vi "4Pi Objective Lock.vi"(7 "Calling VI Ref":refnum<vi>) -> ()   [LabVIEW 2016]
uses:
  <vilib>/Utility/miscctls.llb/LVPointTypeDef.ctl
  4Pi Objective Lock Type Defs/4Pi Obj Lock - Notifier Type.ctl
  4Pi Objective Lock Type Defs/4Pi Obj Lock - Actions.ctl
  4Pi Objective Lock Type Defs/4Pi Obj Lock - Lock Settings.ctl
  Hardware Configuration/Hardware Configuration Controls/Device Type.ctl
  Hardware Configuration/Hardware Configuration Controls/Device Function.ctl
  4Pi Objective Lock Type Defs/4Pi Obj Lock - Camera Settings.ctl
  Device Library/Cameras/Camera Controls/Generic Camera ROI.ctl
  Device Library/Cameras/Camera Controls/Generic Camera Actions.ctl
  Device Library/Stages/Stages Controls/Stage Actions.ctl
  <vilib>/addons/control/pid/pid.llb/PID (DBL Array).vi
  <vilib>/addons/control/pid/NI_PID_pid.lvlib
panel:
  in  "Main Tab":T1(tab)
  out "Z Move":bool
  out "XY Move":bool
  out "Measured X Position (px)":dbl=1.0 format="%.3g"
  out "Measured Y Position (px)":dbl=1.0 format="%.3g"
  out "Measured sx/sy":dbl=1.0 format="%.3g"
  out "Target X Position (px)":dbl=1.0 format="%.3g"
  out "Target Y Position (px)":dbl=1.0 format="%.3g"
  out "Target sx/sy":dbl=1.0 format="%.3g"
  out "Z Axis Position (µm)":dbl=1.0 format="%.4g"
  out "Y Axis Position (µm)":dbl=1.0 format="%.2g"
  out "X Axis Position (µm)":dbl=1.0 format="%.2g"
  out "Z sx/sy Target and Fit Value":T2(graph)
  in  "Start Lock":bool
  out "Y Target and Fit Position (px)":T2(graph)
  out "X Target and Fit Position (px)":T2(graph)
  in  "Restart Lock":bool
  out "Fit Error":bool
  out "Move Limit Error":bool
  in  "Update Delay (ms)":i32=10
  in  "D (Derivative)":dbl
  in  "I (Integral)":dbl
  in  "P (Proportional)":dbl=2.0
  in  "Invert Z Axis":bool
  in  "XY Drift Threshold":dbl=0.05
  in  "Abort If Error":bool
  in  "Flip XY Axis":bool
  in  "Invert X Axis":bool
  in  "Invert Y Axis":bool
  in  "Z Stage Move Limit (µm)":dbl=5.0
  in  "Z Drift Threshold":dbl=0.05
  in  "XY Stage Move Limit (µm)":dbl=1.0
  in  "Frame Accumulations":u16=10
  in  "XY Correction Active":bool=TRUE
  in  "Z Correction Active":bool=TRUE
  in  "Set Camera ROI":bool
  in  "Save Lock Settings":bool
  in  "Quit":bool
  # "Z Drift Settings"
  # "Camera Setup"
  # "XY Drift Settings"
  # "PID Control Values"
  # "General Settings"
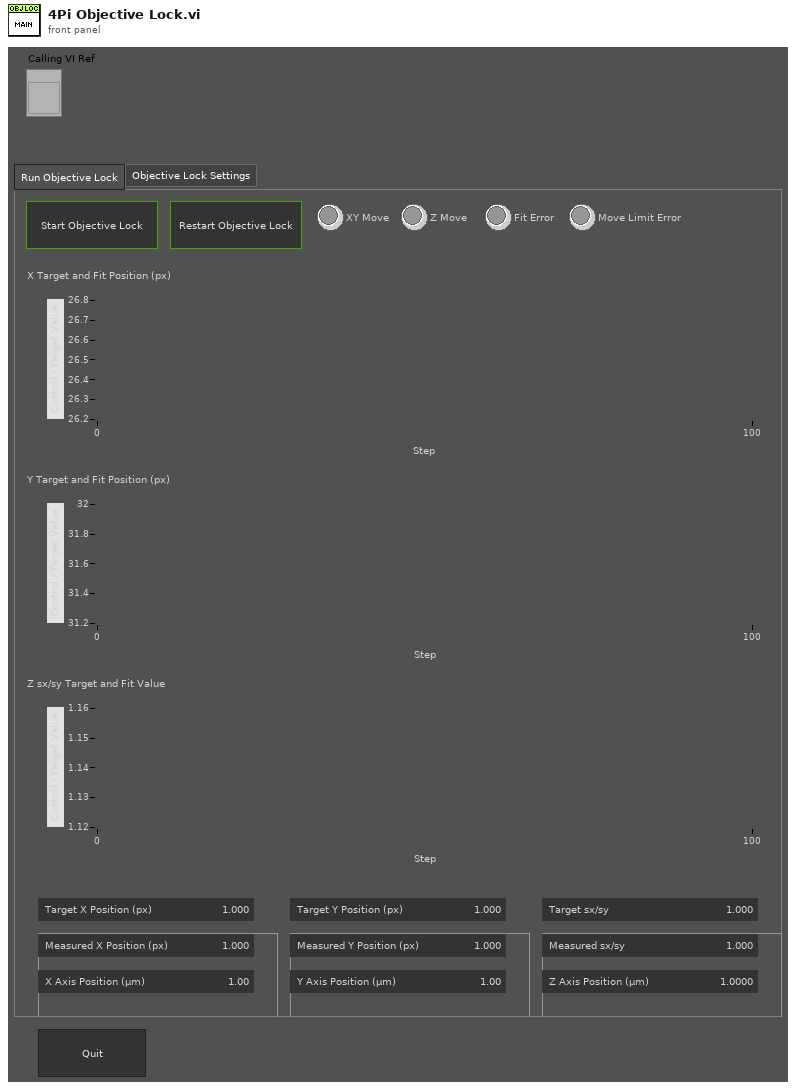
[diagram p1: front panel]
types:
  T1 = enum32{"Run Objective Lock", "Objective Lock Settings"}
  T2 = cluster{"Target 01":dbl, dbl, dbl, "Current 01":dbl}
  T3 = typedef "4Pi Obj Lock - Camera Settings.ctl" = cluster{"Exposure Time (s)":dbl, "H Offset":u16, "V Offset":u16, "H Width":u16, "V Width":u16}
  T4 = typedef "Device Function.ctl" = enum16{"Primary", "Secondary", "Overview", "Wide Field Drift Correction", "642 nm Excitation", "560 nm Excitation", "546 nm Excitation", "488 nm Excitation", "405 nm Excitation", "Objective Drift Correction", "4Pi Objective Lock", "Objective XY", "Objective Z", "Sample XY", "Sample Coarse Z", "Sample Z", "4Pi Lower", "4Pi Upper", "Adj Cavity", "Line Scanning", "Alert"}
  T5 = typedef "Device Type.ctl" = enum16{"AOTF", "Camera", "Deformable Mirror", "Laser", "Shutter", "Stage", "Waveform", "Email"}
  T6 = typedef "4Pi Obj Lock - Actions.ctl" = enum16{"Idle", "Start Lock", "Restart Lock", "Get Initial Position", "Get Current Position", "Check Drift", "Move XYZ", "Move XY", "Move Z", "Update Plots", "Delay", "Abort", "Exit Loop", "Quit"}
  T7 = typedef "4Pi Obj Lock - Lock Settings.ctl" = cluster{"Z Drift Threshold":dbl, "Z Stage Move Limit (µm)":dbl, "XY Drift Threshold":dbl, "XY Stage Move Limit (µm)":dbl, "Frame Accumulations":u16, "Abort If Error":bool, "Flip XY Axis":bool, "Invert X Axis":bool, "Invert Y Axis":bool, "Invert Z Axis":bool, "Z Correction Active":bool, "XY Correction Active":bool, "PID Values":dbl[], "Update Delay (ms)":i32}
  T8 = typedef "4Pi Obj Lock - Notifier Type.ctl" = cluster{"Actions":T6, "Z Drift Threshold":dbl, "Z Stage Move Limit (µm)":dbl, "XY Drift Threshold":dbl, "XY Stage Move Limit (µm)":dbl, "Frame Accumulations":u16, "Abort If Error":bool, "Z Correction Active":bool, "XY Correction Active":bool, "PID Values":dbl[], "Running?":bool, "Update Delay (ms)":i32}
  T9 = enum16{"Always On", "Always Off", "Off While Running"}
  T10 = typedef "LVPointTypeDef.ctl" = cluster{"Horizontal":i16, "Vertical":i16}
  T11 = typedef "Generic Camera Actions.ctl" = enum16{"Status", "Live Preview", "Capture", "Abort", "Set Exposure Time (s)", "Get Exposure Time (s)", "Record Settings", "Set ROI", "Get ROI", "Defect Correction On/Off", "Cooler On/Off", "Fan On/Off", "Quti"}
  T12 = typedef "Generic Camera ROI.ctl" = cluster{"H_Offset":u16, "V_Offset":u16, "H_Width":u16, "V_Width":u16}
  T13 = typedef "Stage Actions.ctl" = enum16{"Get Position", "MVR", "MOVE", "HALT", "ONTARGET", "ERROR", "REFERENCE", "INIT", "VELOCITY", "STATUS", "EXIT", "HOME", "ZEROPOS", "NANOPOS", "ANALOG", "QUIT"}
  T14 = enum32{"Invalid", "Standard", "Closed", "Hidden", "Minimized", "Maximized"}
  T15 = cluster{"Target 01":dbl, dbl, dbl, "Current 01":dbl}[]
  T16 = typedef "2D Gaussian - Best Fit Parameters.ctl" = cluster{"Amplitude":dbl, "X Position":dbl, "Y Position":dbl, "X Width":dbl, "Y Width":dbl, "Offset":dbl}
  T17 = cluster{"PID Values[0]":dbl, "PID Values[1]":dbl, "PID Values[2]":dbl}
  T18 = cluster{"PID Values[0]":dbl, "PID Values[1]":dbl, "PID Values[2]":dbl}[]
  T19 = typedef "LVRectTypeDef.ctl" = cluster{"Left":i16, "Top":i16, "Right":i16, "Bottom":i16}
  T20 = typedef "LVBoundsTypeDef.ctl" = cluster{"Width":u32, "Height":u32}
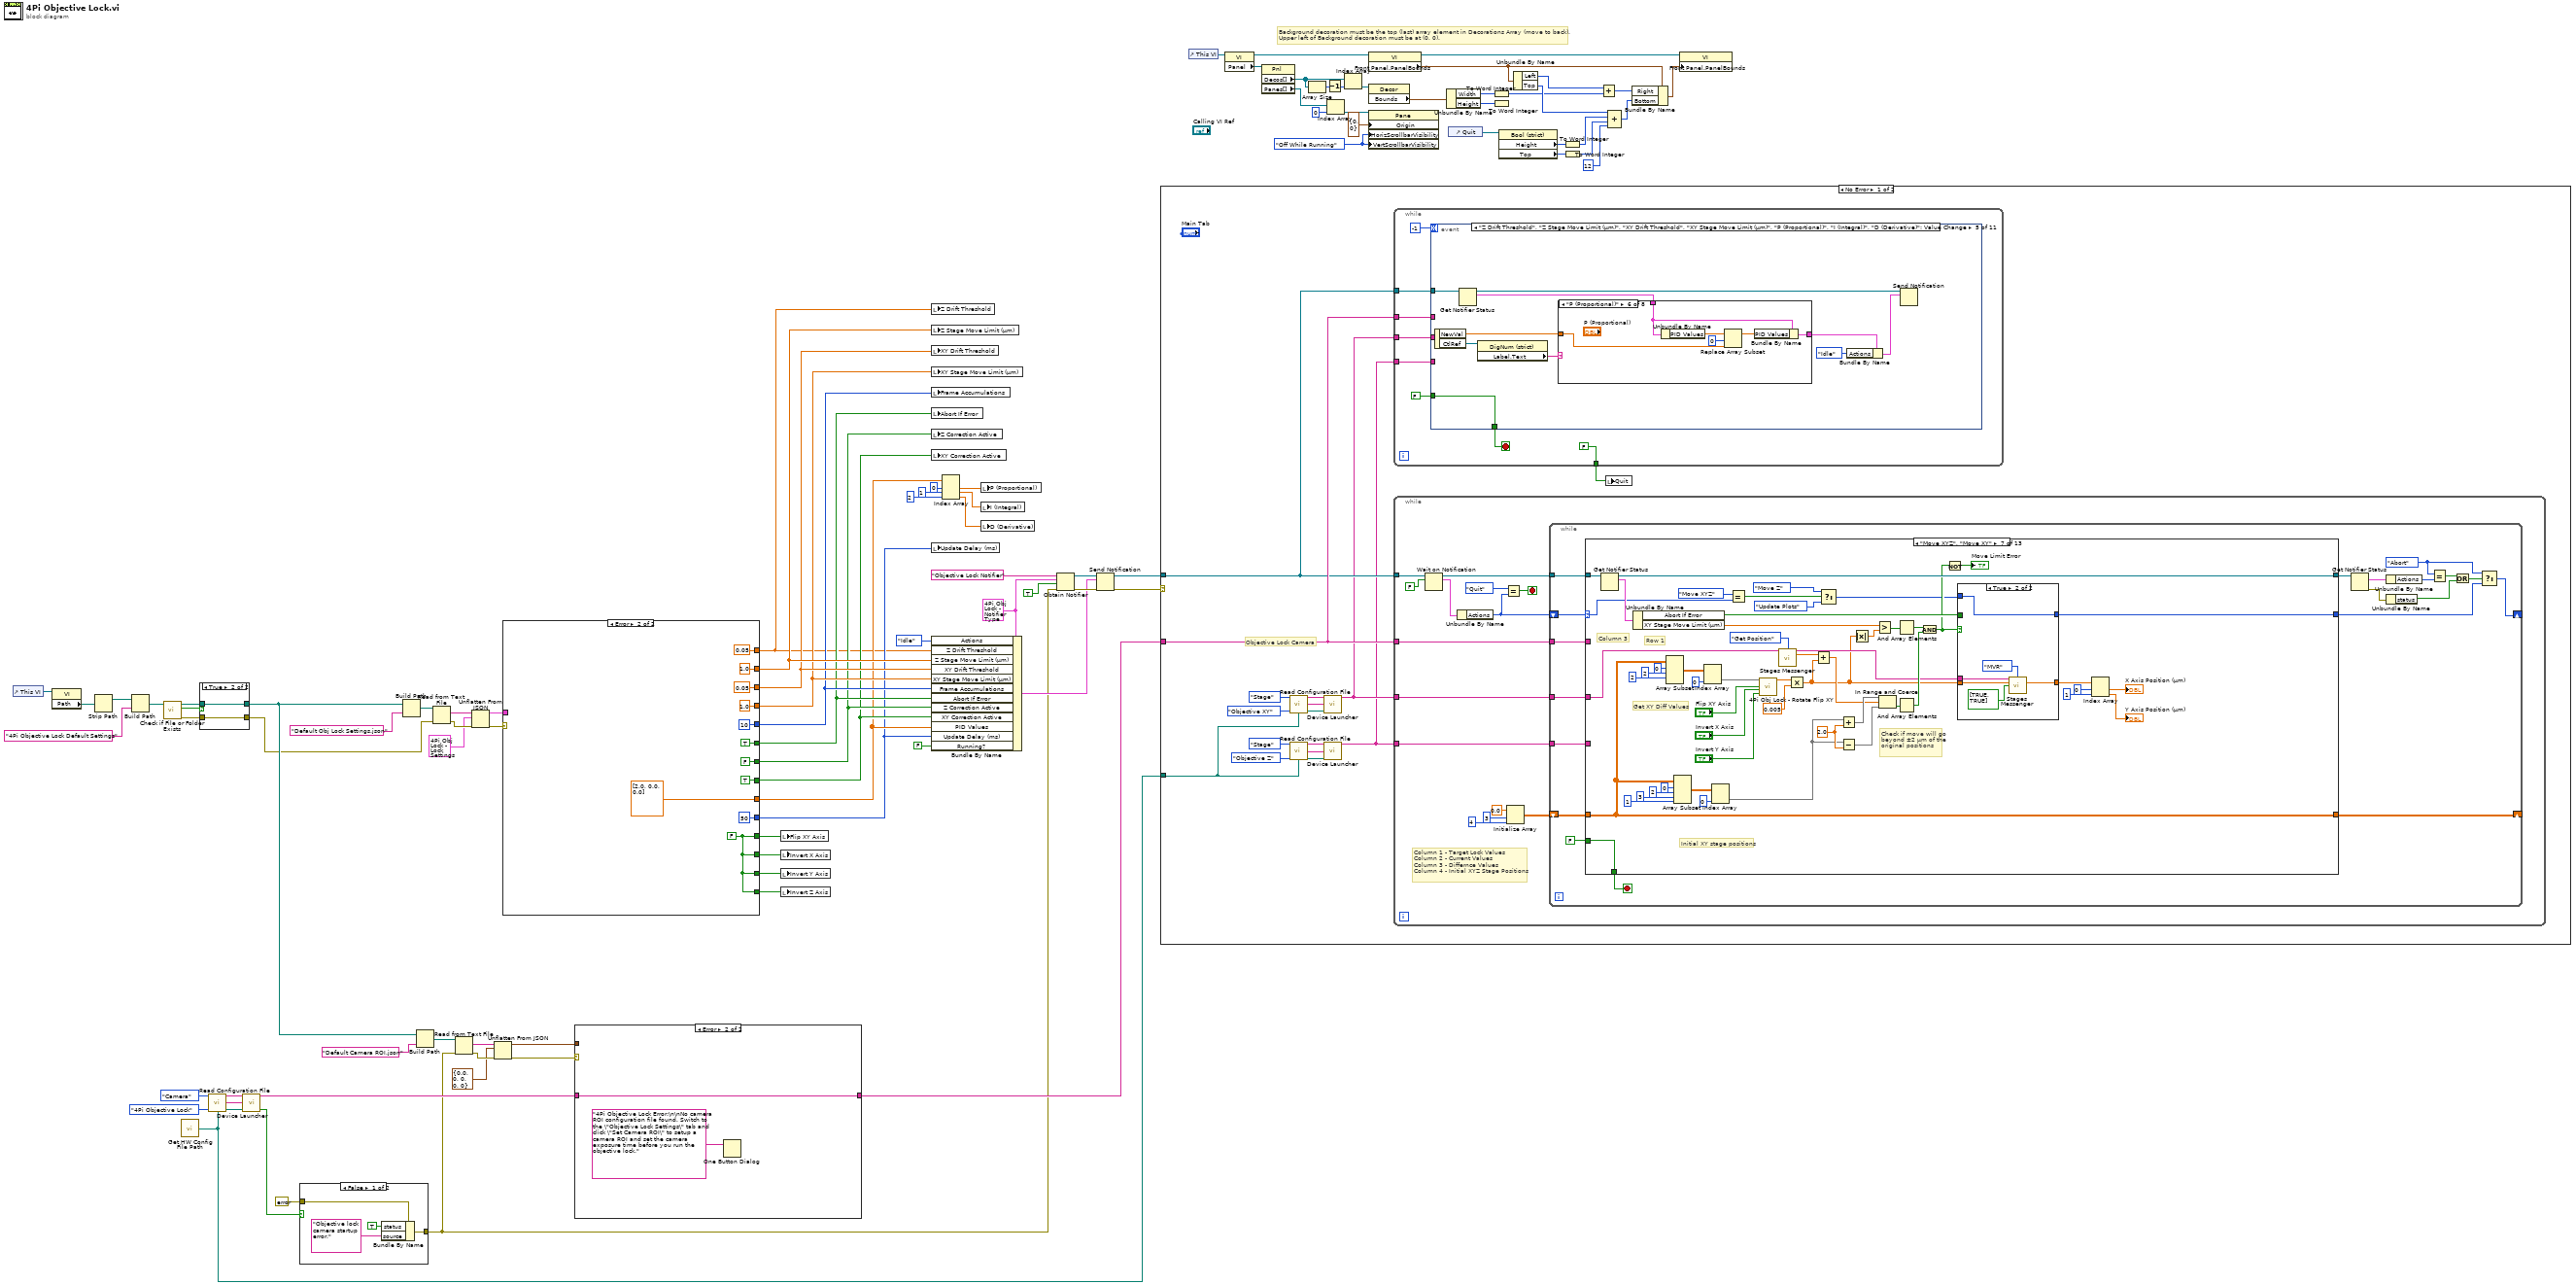
[diagram p0: block diagram]
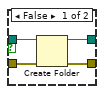
[diagram p2: hidden frame]
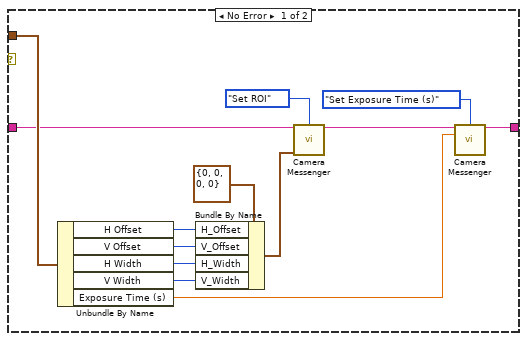
[diagram p4: hidden frame]
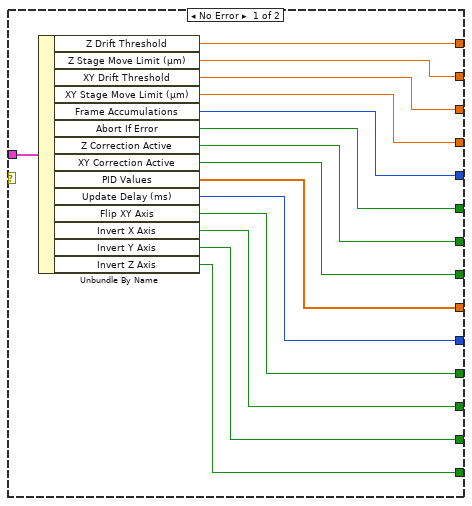
[diagram p5: hidden frame]
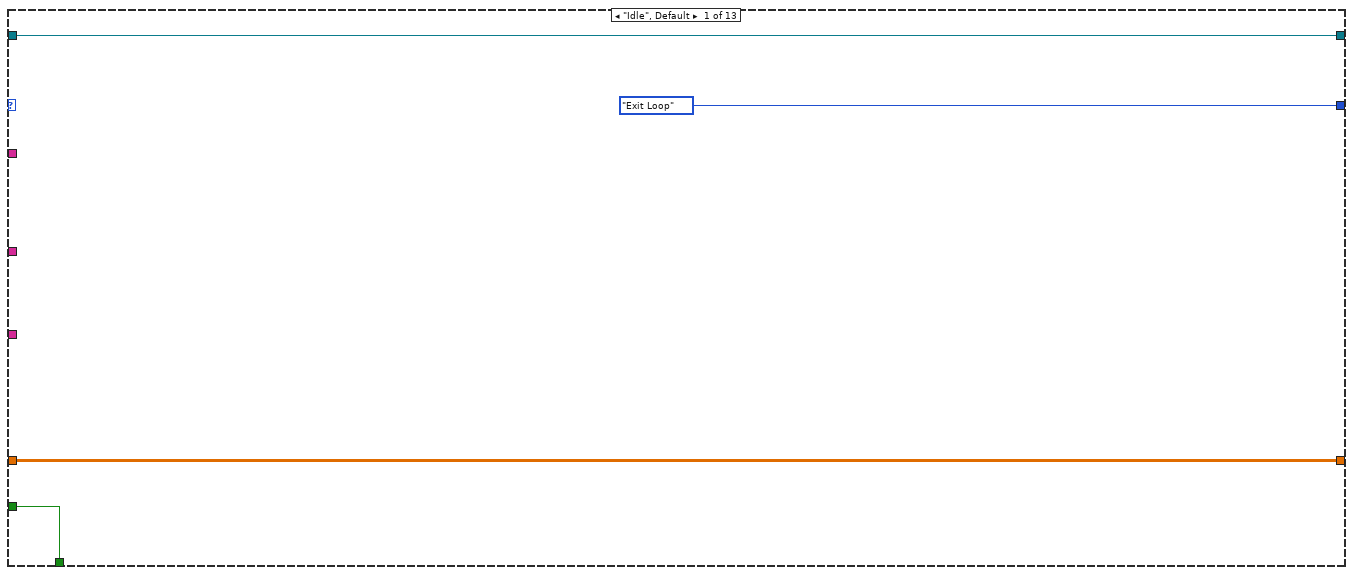
[diagram p6: hidden frame]
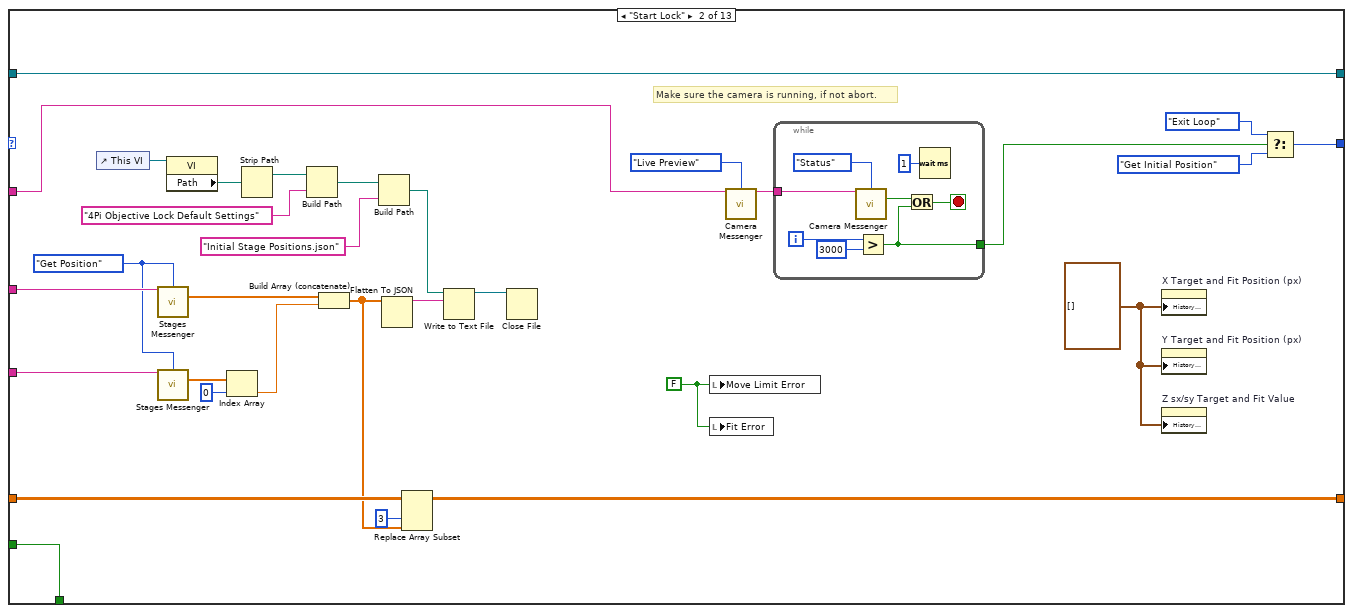
[diagram p7: hidden frame]
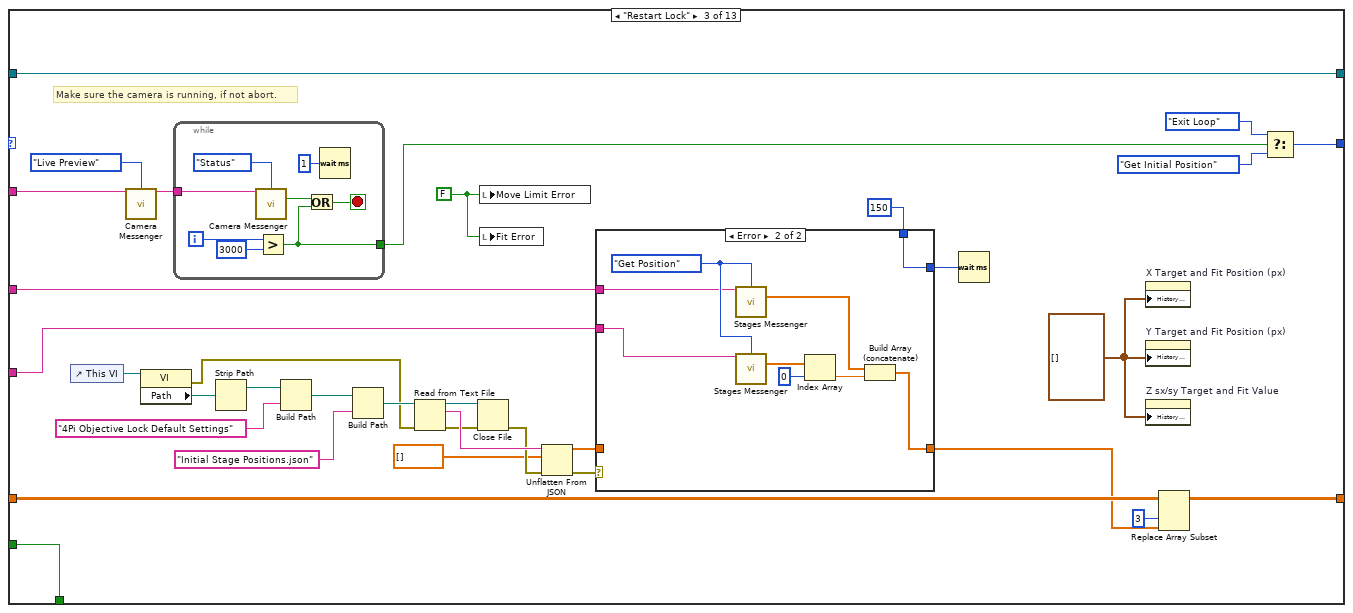
[diagram p8: hidden frame]
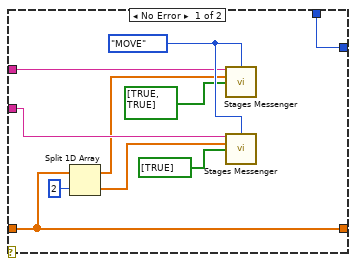
[diagram p9: hidden frame]
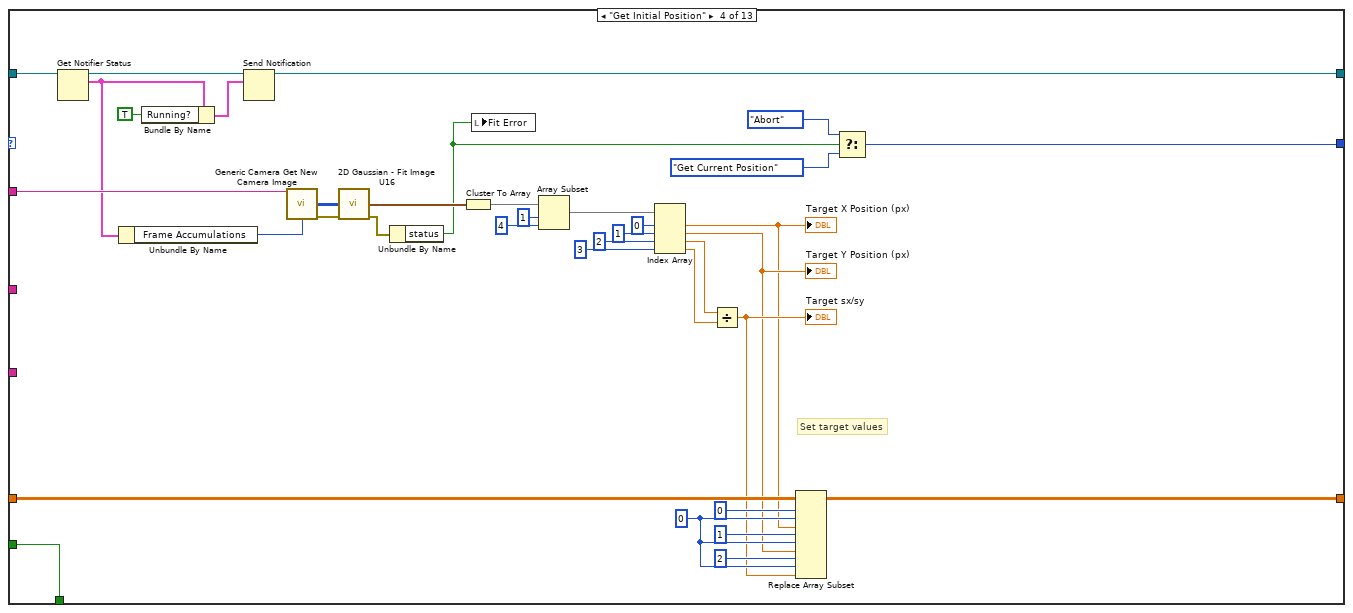
[diagram p10: hidden frame]
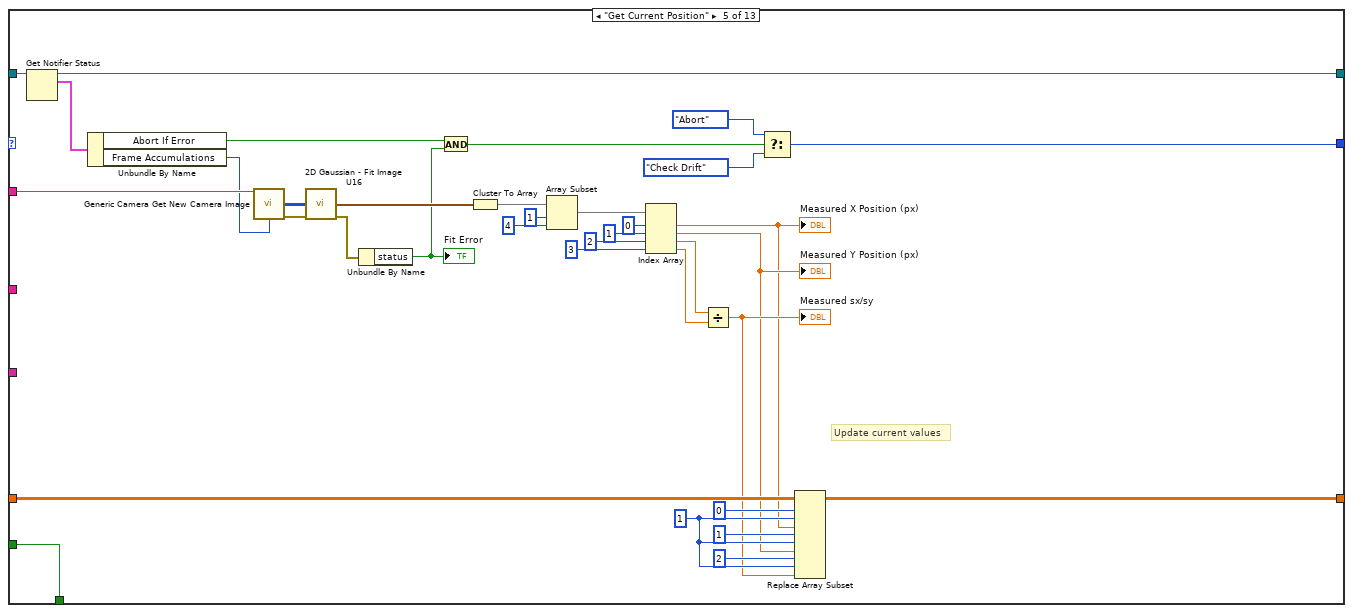
[diagram p11: hidden frame]
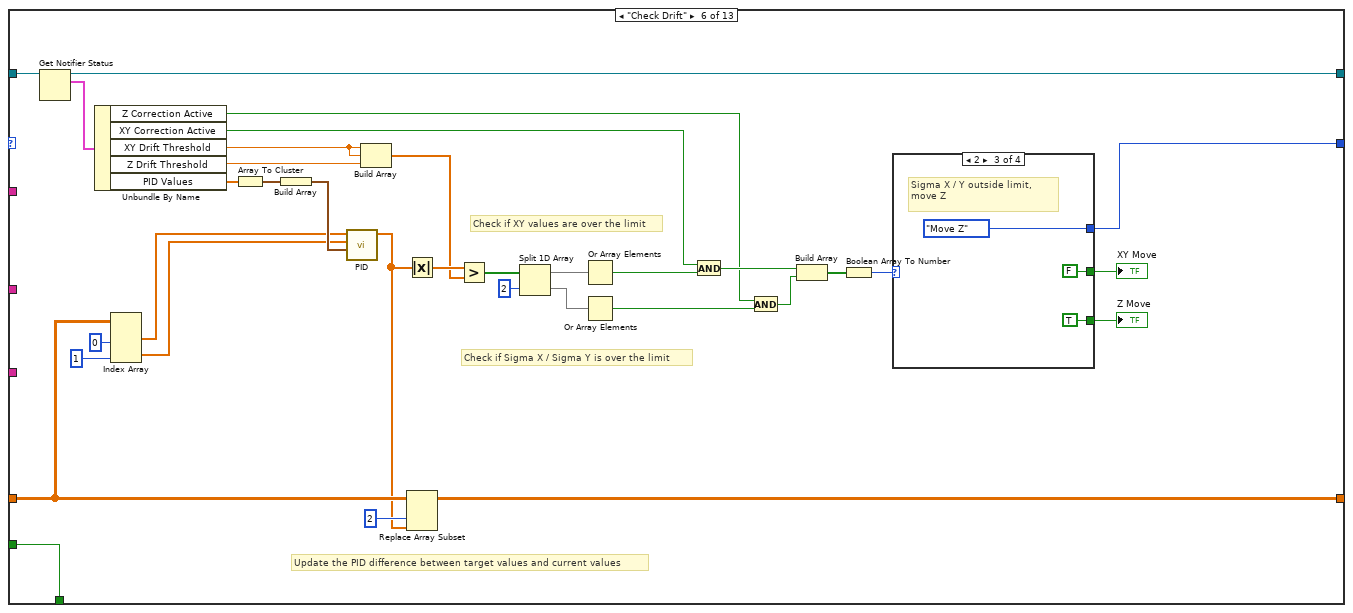
[diagram p12: hidden frame]
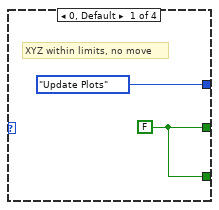
[diagram p13: hidden frame]
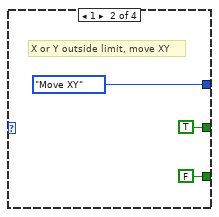
[diagram p14: hidden frame]
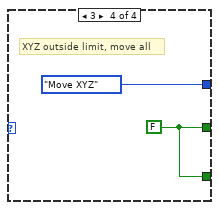
[diagram p15: hidden frame]
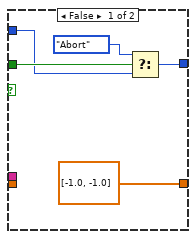
[diagram p16: hidden frame]
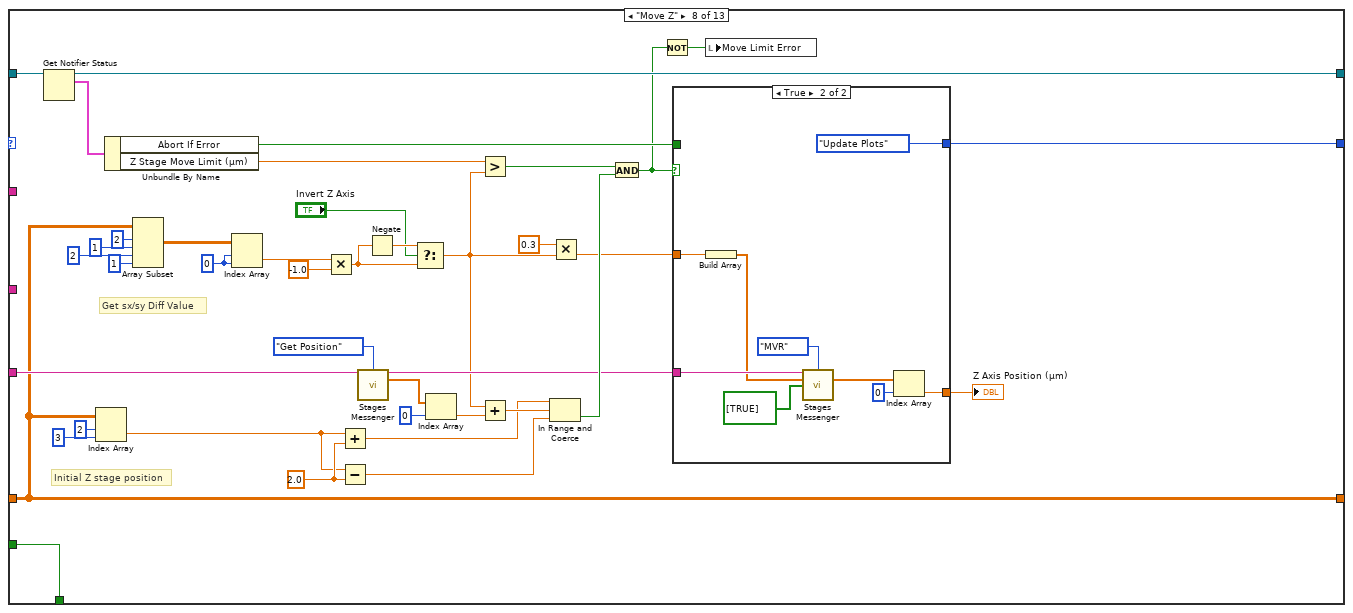
[diagram p17: hidden frame]
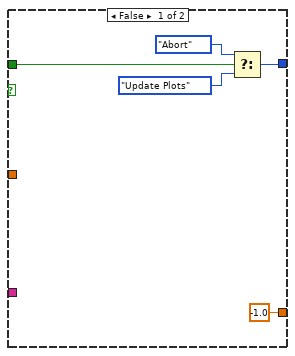
[diagram p18: hidden frame]
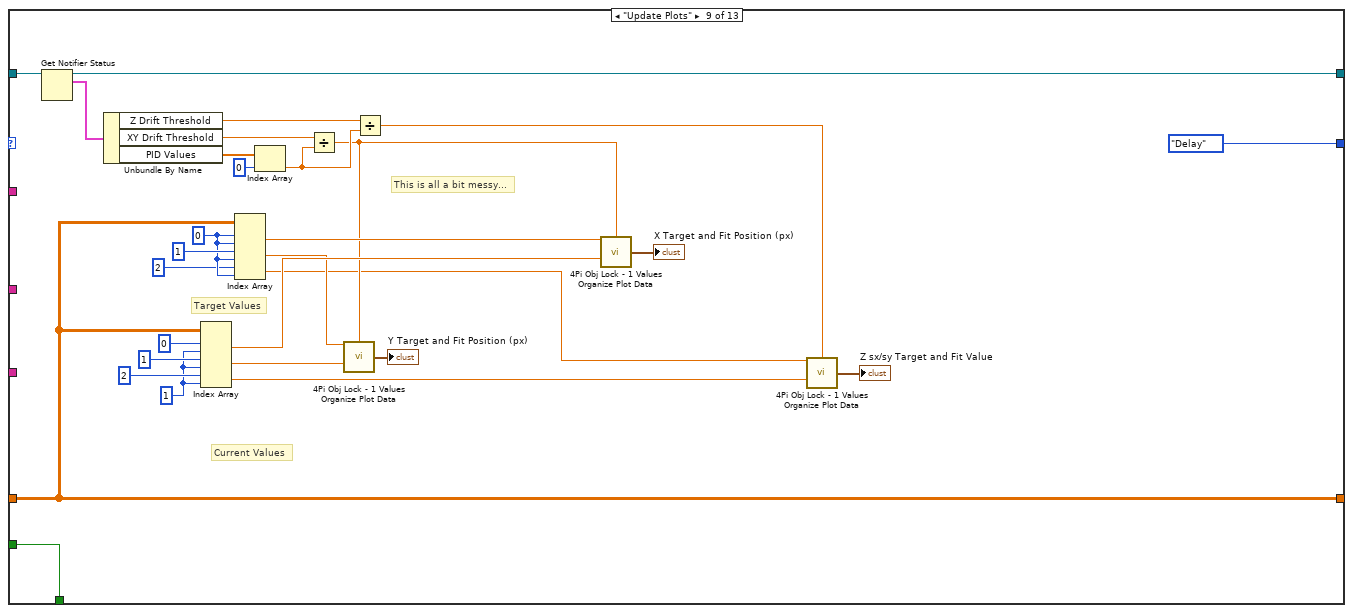
[diagram p19: hidden frame]
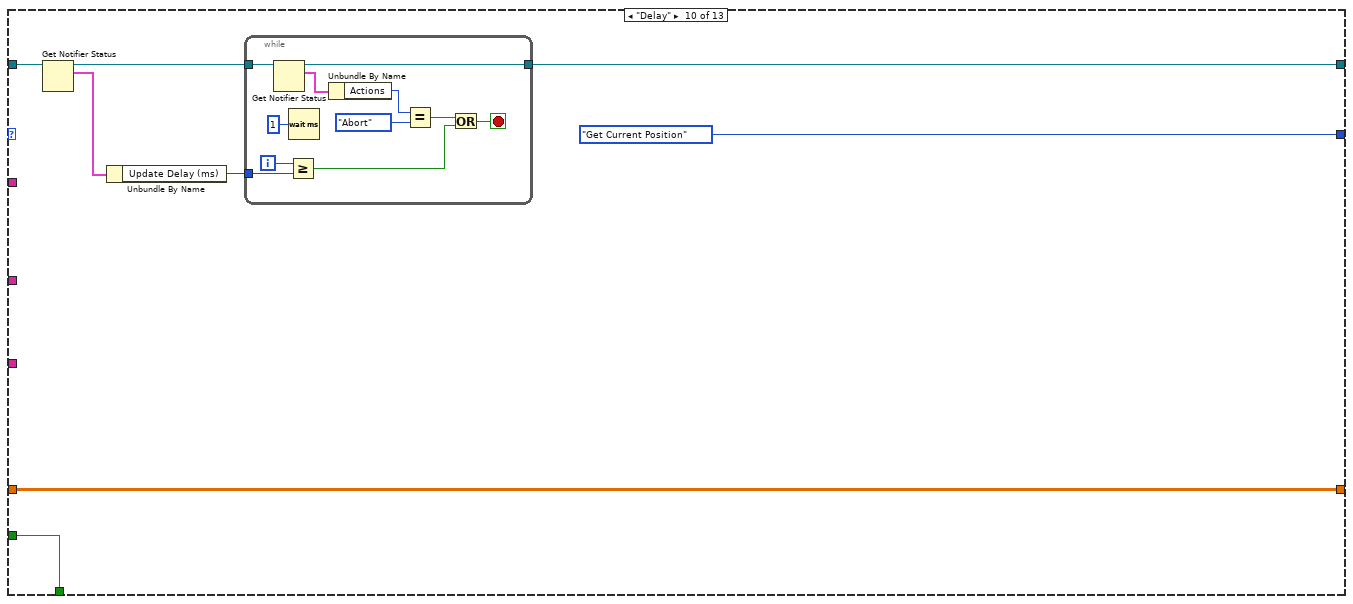
[diagram p20: hidden frame]
diagram:
  w60 = T8 {"Actions"=enum."Idle", "Z Drift Threshold"=0.05, "Z Stage Move Limit (µm)"=1.0, "XY Drift Threshold"=0.05, "XY Stage Move Limit (µm)"=1.0, "Frame Accumulations"=10, "Abort If Error"=FALSE, "Z Correction Active"=FALSE, "XY Correction Active"=FALSE, "PID Values"=[], "Running?"=FALSE, "Update Delay (ms)"=0} ("4Pi Obj Lock")
  w77 = T9."Off While Running" ("Vertical Scrollbar Visibility")
  # "Background decoration must be the top (last) array element in Decorations Array (move to back).\nUpper left of Background decoration must be at (0, 0)."
  n1 = control-ref of="This VI"() -> (w48:refnum<vi>)
  n2 = property class="VI"(reference=w48) -> ("Path"=w30:path)  [unwired: 1 in, 2 out]
  n3 = Strip Path(path=w30) -> (stripped path=w29:path)  [unwired: 1 out]
  n4 = Build Path(base path=w29, name or relative path="4Pi Objective Lock Default Settings") -> (appended path=w6:path)
  n5 = call <vilib>:"Check if File or Folder Exists.vi"("path"=w6) -> ("error out"=w2:errorcluster, "file or folder exists?"=w5:bool, "dup path"=w4:path)  [unwired: 8 in]
  n6 = call "Get HW Config File Path.vi"() -> ("File Path"=w38:path)  [unwired: 14 in, 1 out]
  n7 = case shown="True" w5 {
    tunnel: w4 -> [w98 w100]
    tunnel: [w97 w100] -> w3
    tunnel: w2 -> [w96 w99]
    tunnel: [w95 w99] -> w1
    frame False {
      n8 = Create Folder(path (use dialog)=w98, error in=w96) -> (created path=w97:path, error out=w95:errorcluster)  [unwired: 1 in, 1 out]
    }
    frame True {
    }
  }
  n9 = call "Read Configuration File.vi"("Device Type"=Device_Type."Camera", "Device Function"=Device_Function."4Pi Objective Lock", "Config File Path"=w38) -> ("Unique Notifier Name"=w45:string, "Device Ports/IDs/Channels"=w47:string[], "Device Engine Path"=w46:path)  [unwired: 9 in, 1 out]
  n10 = call "Device Launcher.vi"("Notifier Name"=w45, "Device Ports/IDs/Channels"=w47, "Device Engine Path"=w46) -> ("Notifier Name"=w36:string, "Running?"=w42:bool)  [unwired: 11 in]
  n11 = case shown="False" w42 {
    tunnel: errorcluster {"status"=FALSE, "code"=0, "source"=""} ("Error") -> [w104 w105]
    tunnel: [w101 w105] -> w28
    frame False {
      n12 = Bundle By Name(cluster=w104, "status"=TRUE, "source"="Objective lock camera startup error." ("name or relative path")) -> (w101:errorcluster)
    }
    frame True {
    }
  }
  n13 = Build Path(base path=w3, name or relative path="Default Obj Lock Settings.json") -> (appended path=w57:path)
  n14 = Build Path(base path=w3, name or relative path="Default Camera ROI.json") -> (appended path=w32:path)
  n15 = Read from Text File(file (use dialog)=w57, error in=w1) -> (text=w56:string, error out=w55:errorcluster)  [unwired: 2 in, 2 out]
  n16 = Read from Text File(file (use dialog)=w32, error in=w28) -> (text=w50:string, error out=w49:errorcluster)  [unwired: 2 in, 2 out]
  n17 = Unflatten From JSON(JSON string=w56, type and defaults=T7 {"Z Drift Threshold"=0.05, "Z Stage Move Limit (µm)"=1.0, "XY Drift Threshold"=0.05, "XY Stage Move Limit (µm)"=1.0, "Frame Accumulations"=10, "Abort If Error"=FALSE, "Flip XY Axis"=FALSE, "Invert X Axis"=FALSE, "Invert Y Axis"=FALSE, "Invert Z Axis"=FALSE, "Z Correction Active"=TRUE, "XY Correction Active"=TRUE, "PID Values"=[], "Update Delay (ms)"=0} ("Lock Settings"), error in (no error)=w55) -> (value=w52:T7, error out=w53:errorcluster)  [unwired: 4 in]
  n18 = Unflatten From JSON(JSON string=w50, type and defaults=T3 {"Exposure Time (s)"=0.0, "H Offset"=0, "V Offset"=0, "H Width"=0, "V Width"=0} ("Camera Settings"), error in (no error)=w49) -> (value=w35:T3, error out=w40:errorcluster)  [unwired: 4 in]
  n19 = case shown="Error" w53 {
    tunnel: [w119 0.05 ("Z Drift Threshold")] -> w7
    tunnel: [w118 1.0 ("Z Stage Move Limit (µm)")] -> w22
    tunnel: [w116 0.05 ("XY Drift Threshold")] -> w21
    tunnel: [w117 1.0 ("XY Stage Move Limit (µm)")] -> w20
    tunnel: [w115 u16 10 ("Frame Accumulations")] -> w19
    tunnel: [w114 TRUE ("Abort If Error")] -> w18
    tunnel: w52 -> [w120 _]
    tunnel: [w113 FALSE ("Z Correction Active")] -> w17
    tunnel: [w112 TRUE ("XY Correction Active")] -> w16
    tunnel: [w111 dbl[] [2.0, 0.0, 0.0] ("PID Values")] -> w15
    tunnel: [w110 u16 50 ("Update Delay (ms)")] -> w8
    tunnel: [w109 w121] -> w24
    tunnel: [w108 w121] -> w25
    tunnel: [w107 w121] -> w26
    tunnel: [w106 w121] -> w27
    frame No Error {
      n20 = Unbundle By Name(w120) -> ("Z Drift Threshold"=w119:dbl, "Z Stage Move Limit (µm)"=w118:dbl, "XY Drift Threshold"=w116:dbl, "XY Stage Move Limit (µm)"=w117:dbl, "Frame Accumulations"=w115:u16, "Abort If Error"=w114:bool, "Z Correction Active"=w113:bool, "XY Correction Active"=w112:bool, "PID Values"=w111:dbl[], "Update Delay (ms)"=w110:i32, "Flip XY Axis"=w106:bool, "Invert X Axis"=w107:bool, "Invert Y Axis"=w108:bool, "Invert Z Axis"=w109:bool)
    }
    frame Error {
      w121 = FALSE ("Flip XY Axis")
    }
  }
  n21 = case shown="Error" w40 {
    tunnel: w36 -> [w135 w146]
    tunnel: w35 -> [w144 _]
    tunnel: [w132 w146] -> w34
    frame No Error {
      n22 = Unbundle By Name(w144) -> ("H Offset"=w139:u16, "V Offset"=w140:u16, "H Width"=w141:u16, "V Width"=w142:u16, "Exposure Time (s)"=w134:dbl)
      n23 = Bundle By Name(cluster=T12 {"H_Offset"=0, "V_Offset"=0, "H_Width"=0, "V_Width"=0} ("General Camera ROI"), "H_Offset"=w139, "V_Offset"=w140, "H_Width"=w141, "V_Width"=w142) -> (w138:T12)
      n24 = call "Camera Messenger.vi"("Notifier Name"=w135, "General Camera Actions"=Generic_Camera_Actions."Set ROI", "Camera ROI"=w138) -> ("Notifier Name Dup"=w133:string)  [unwired: 7 in, 5 out]
      n25 = call "Camera Messenger.vi"("Notifier Name"=w133, "General Camera Actions"=Generic_Camera_Actions."Set Exposure Time (s)", "Exposure Time (s)"=w134) -> ("Notifier Name Dup"=w132:string)  [unwired: 7 in, 5 out]
    }
    frame Error {
      n26 = One Button Dialog(message="4Pi Objective Lock Error:\n\nNo camera ROI configuration file found. Switch to the \"Objective Lock Settings\" tab and click \"Set Camera ROI\" to setup a camera ROI and set the camera exposure time before you run the objective lock.") -> ()  [unwired: 1 in, 1 out]
    }
  }
  n27 = local write "Flip XY Axis"(w27) -> ()
  n28 = local write "Invert X Axis"(w26) -> ()
  n29 = local write "Invert Y Axis"(w25) -> ()
  n30 = local write "Invert Z Axis"(w24) -> ()
  n31 = Bundle By Name(cluster=w60, "Actions"=4Pi_Obj_Lock_-_Actions."Idle", "Z Drift Threshold"=w7, "Z Stage Move Limit (µm)"=w22, "XY Drift Threshold"=w21, "XY Stage Move Limit (µm)"=w20, "Frame Accumulations"=w19, "Abort If Error"=w18, "Z Correction Active"=w17, "XY Correction Active"=w16, "PID Values"=w15, "Update Delay (ms)"=w8, "Running?"=FALSE ("Obj Lock Active?")) -> (w59:T8)
  n32 = local write "Z Drift Threshold"(w7) -> ()
  n33 = local write "Z Stage Move Limit (µm)"(w22) -> ()
  n34 = local write "XY Drift Threshold"(w21) -> ()
  n35 = local write "XY Stage Move Limit (µm)"(w20) -> ()
  n36 = local write "Frame Accumulations"(w19) -> ()
  n37 = local write "Abort If Error"(w18) -> ()
  n38 = local write "Z Correction Active"(w17) -> ()
  n39 = local write "XY Correction Active"(w16) -> ()
  n40 = local write "Update Delay (ms)"(w8) -> ()
  n41 = Index Array(array=w15, index #1=0 ("index"), index #2=1 ("index"), index #3=2 ("index")) -> (element #1=w11:dbl, element #2=w9:dbl, element #3=w10:dbl)
  n42 = local write "P (Proportional)"(w11) -> ()
  n43 = local write "I (Integral)"(w9) -> ()
  n44 = local write "D (Derivative)"(w10) -> ()
  n45 = Obtain Notifier(name (unnamed)="Objective Lock Notifier", notification data type=w60, create if not found? (T)=TRUE, error in (no error)=w28) -> (notifier out=w62:refnum<notifier>, error out=w63:errorcluster)  [unwired: 1 out]
  n46 = Send Notification(notification=w59, notifier=w62, error in (no error)=w63) -> (notifier out=w61:refnum<notifier>, error out=w39:errorcluster)
  n47 = case shown="No Error" w39 {
    tunnel: w38 -> [w151 _]
    tunnel: w61 -> [w149 _]
    tunnel: w34 -> [w150 _]
    frame No Error {
      # "Objective Lock Camera"
      n48 = call "Read Configuration File.vi"("Device Type"=Device_Type."Stage", "Device Function"=Device_Function."Objective XY", "Config File Path"=w151) -> ("Unique Notifier Name"=w159:string, "Device Ports/IDs/Channels"=w157:string[], "Device Engine Path"=w158:path)  [unwired: 9 in, 1 out]
      n49 = call "Read Configuration File.vi"("Device Type"=Device_Type."Stage", "Device Function"=Device_Function."Objective Z", "Config File Path"=w151) -> ("Unique Notifier Name"=w154:string, "Device Ports/IDs/Channels"=w156:string[], "Device Engine Path"=w155:path)  [unwired: 9 in, 1 out]
      n50 = call "Device Launcher.vi"("Notifier Name"=w159, "Device Ports/IDs/Channels"=w157, "Device Engine Path"=w158) -> ("Notifier Name"=w148:string)  [unwired: 11 in, 1 out]
      n51 = call "Device Launcher.vi"("Notifier Name"=w154, "Device Ports/IDs/Channels"=w156, "Device Engine Path"=w155) -> ("Notifier Name"=w147:string)  [unwired: 11 in, 1 out]
      n52 = while {
        tunnel: [FALSE] -> w162
        tunnel: w150 -> [w607]
        tunnel: w149 -> [w606]
        tunnel: w148 -> [w605]
        tunnel: w147 -> [w604]
        stop <- w609 stop-if-true
        n53 = event shown="[4] \"Z Drift Threshold\", \"Z Stage Move Limit (µm)\", \"XY Drift Threshold\", \"XY Stage Move Limit (µm)\", \"P (Proportional)\", \"I (Integral)\", \"D (Derivative)\": Value Change" {
          selector: _ -> [_ _ _ _ _ _ _ _ _ _ _]
          dyn-events: _ -> [_ _ _ _ _ _ _ _ _ _ _]
          timeout: -1 -> [_ _ _ _ _ _ _ _ _ _ _]
          tunnel: FALSE -> [w612 w616 w619 w629 w649 w687 w694 w721 w730 w737 _]
          tunnel: [w612 w616 w619 w629 w649 w687 w694 w721 w730 w737 w747] -> w609
          tunnel: w607 -> [_ _ w618 _ _ _ _ _ _ _ _]
          tunnel: w606 -> [_ _ _ w628 w646 w686 w693 w720 w729 w736 w742]
          tunnel: w605 -> [_ _ _ _ _ _ _ _ _ _ _]
          tunnel: w604 -> [_ _ _ _ _ _ _ _ _ _ _]
          event Timeout {
            n54 = event-data() -> ()  [unwired: 1 in, 1 out]
          }
          event Application Instance Close? {
            n55 = event-data() -> ()  [unwired: 1 in, 1 out]
            n56 = control-ref of="This VI"() -> (w613:refnum<vi>)
            n57 = invoke class="VI" method="FP.Open"(reference=w613, "Activate"=TRUE ("Activate?"), "State"=T14."Standard") -> ()  [unwired: 2 in, 5 out]
            n58 = event-data("Discard?"=TRUE) -> ()  [unwired: 1 in, 1 out]
          }
          event "Set Camera ROI": Value Change {
            n59 = event-data() -> ()  [unwired: 1 in, 2 out]
            n60 = call "4Pi Obj Lock - Setup Camera.vi"("Camera Notifier Name"=w618) -> ()  [unwired: 14 in, 1 out]
          }
          event "XY Correction Active", "Z Correction Active", "Abort If Error": Value Change {
            n61 = event-data() -> ("NewVal"=w624:bool, "CtlRef"=w627:refnum<vi>)  [unwired: 1 in]
            n62 = Get Notifier Status(notifier=w628) -> (notifier out=w626:refnum<notifier>, current notification=w623:T8)  [unwired: 1 in, 3 out]
            n63 = property class="Bool (strict)"(reference=w627) -> ("Label.Text"=w625:string)  [unwired: 1 in, 2 out]
            n64 = case shown="\"XY Correction Active\"" w625 {
              tunnel: w624 -> [_ w632 w635 w638]
              tunnel: w623 -> [w630 w633 w636 w639]
              tunnel: [w630 w631 w634 w637] -> w622
              frame Default {
              }
              frame "XY Correction Active" {
                n65 = Bundle By Name(cluster=w633, "XY Correction Active"=w632) -> (w631:T8)
              }
              frame "Z Correction Active" {
                n66 = Bundle By Name(cluster=w636, "Z Correction Active"=w635) -> (w634:T8)
              }
              frame "Abort If Error" {
                n67 = Bundle By Name(cluster=w639, "Abort If Error"=w638) -> (w637:T8)
              }
            }
            n68 = Bundle By Name(cluster=w622, "Actions"=4Pi_Obj_Lock_-_Actions."Idle") -> (w620:T8)
            n69 = Send Notification(notification=w620, notifier=w626) -> ()  [unwired: 1 in, 2 out]
          }
          event "Z Drift Threshold", "Z Stage Move Limit (µm)", "XY Drift Threshold", "XY Stage Move Limit (µm)", "P (Proportional)", "I (Integral)", "D (Derivative)": Value Change {
            n70 = event-data() -> ("NewVal"=w644:dbl, "CtlRef"=w645:refnum<vi>)  [unwired: 1 in]
            n71 = Get Notifier Status(notifier=w646) -> (notifier out=w643:refnum<notifier>, current notification=w647:T8)  [unwired: 1 in, 3 out]
            n72 = property class="DigNum (strict)"(reference=w645) -> ("Label.Text"=w648:string)  [unwired: 1 in, 2 out]
            n73 = case shown="\"P (Proportional)\"" w648 {
              tunnel: w644 -> [_ w652 w655 w658 w661 w666 w672 w678]
              tunnel: w647 -> [w650 w653 w656 w659 w662 w665 w671 w677]
              tunnel: [w650 w651 w654 w657 w660 w663 w669 w675] -> w641
              frame Default {
              }
              frame "Z Drift Threshold" {
                n74 = Bundle By Name(cluster=w653, "Z Drift Threshold"=w652) -> (w651:T8)
              }
              frame "Z Stage Move Limit (µm)" {
                n75 = Bundle By Name(cluster=w656, "Z Stage Move Limit (µm)"=w655) -> (w654:T8)
              }
              frame "XY Drift Threshold" {
                n76 = Bundle By Name(cluster=w659, "XY Drift Threshold"=w658) -> (w657:T8)
              }
              frame "XY Stage Move Limit (µm)" {
                n77 = Bundle By Name(cluster=w662, "XY Stage Move Limit (µm)"=w661) -> (w660:T8)
              }
              frame "P (Proportional)" {
                n78 = Unbundle By Name(w665) -> ("PID Values"=w668:dbl[])
                n79 = Replace Array Subset(array=w668, new element=w666, index=0) -> (w664:dbl[])
                n80 = Bundle By Name(cluster=w665, "PID Values"=w664) -> (w663:T8)
              }
              frame "I (Integral)" {
                n81 = Unbundle By Name(w671) -> ("PID Values"=w674:dbl[])
                n82 = Replace Array Subset(array=w674, new element=w672, index=1) -> (w670:dbl[])
                n83 = Bundle By Name(cluster=w671, "PID Values"=w670) -> (w669:T8)
              }
              frame "D (Derivative)" {
                n84 = Unbundle By Name(w677) -> ("PID Values"=w680:dbl[])
                n85 = Replace Array Subset(array=w680, new element=w678, index=2) -> (w676:dbl[])
                n86 = Bundle By Name(cluster=w677, "PID Values"=w676) -> (w675:T8)
              }
            }
            n87 = Bundle By Name(cluster=w641, "Actions"=4Pi_Obj_Lock_-_Actions."Idle") -> (w640:T8)
            n88 = Send Notification(notification=w640, notifier=w643) -> ()  [unwired: 1 in, 2 out]
          }
          event "Frame Accumulations": Value Change {
            n89 = event-data() -> ("NewVal"=w683:u16)  [unwired: 1 in]
            n90 = Get Notifier Status(notifier=w686) -> (notifier out=w685:refnum<notifier>, current notification=w684:T8)  [unwired: 1 in, 3 out]
            n91 = Bundle By Name(cluster=w684, "Actions"=4Pi_Obj_Lock_-_Actions."Idle", "Frame Accumulations"=w683) -> (w682:T8)
            n92 = Send Notification(notification=w682, notifier=w685) -> ()  [unwired: 1 in, 2 out]
          }
          event "Update Delay (ms)": Value Change {
            n93 = event-data() -> ("NewVal"=w690:i32)  [unwired: 1 in]
            n94 = Get Notifier Status(notifier=w693) -> (notifier out=w692:refnum<notifier>, current notification=w691:T8)  [unwired: 1 in, 3 out]
            n95 = Bundle By Name(cluster=w691, "Actions"=4Pi_Obj_Lock_-_Actions."Idle", "Update Delay (ms)"=w690) -> (w689:T8)
            n96 = Send Notification(notification=w689, notifier=w692) -> ()  [unwired: 1 in, 2 out]
          }
          event "Save Lock Settings": Value Change {
            n97 = event-data() -> ()  [unwired: 1 in, 1 out]
            n98 = Wait on Notification(notifier=w720) -> (notification=w718:T8)  [unwired: 3 in, 3 out]
            n99 = Unbundle By Name(w718) -> ("Z Drift Threshold"=w717:dbl, "Z Stage Move Limit (µm)"=w716:dbl, "XY Drift Threshold"=w715:dbl, "XY Stage Move Limit (µm)"=w714:dbl, "Frame Accumulations"=w713:u16, "Abort If Error"=w712:bool, "Z Correction Active"=w711:bool, "XY Correction Active"=w710:bool, "PID Values"=w700:dbl[])
            n100 = local read "Invert X Axis"() -> (w698:bool)
            n101 = local read "Invert Y Axis"() -> (w697:bool)
            n102 = local read "Invert Z Axis"() -> (w696:bool)
            n103 = local read "Flip XY Axis"() -> (w699:bool)
            n104 = Bundle By Name(cluster=T7 {"Z Drift Threshold"=0.05, "Z Stage Move Limit (µm)"=1.0, "XY Drift Threshold"=0.05, "XY Stage Move Limit (µm)"=1.0, "Frame Accumulations"=10, "Abort If Error"=FALSE, "Flip XY Axis"=FALSE, "Invert X Axis"=FALSE, "Invert Y Axis"=FALSE, "Invert Z Axis"=FALSE, "Z Correction Active"=TRUE, "XY Correction Active"=TRUE, "PID Values"=[], "Update Delay (ms)"=0} ("Lock Settings"), "Z Drift Threshold"=w717, "Z Stage Move Limit (µm)"=w716, "XY Drift Threshold"=w715, "XY Stage Move Limit (µm)"=w714, "Frame Accumulations"=w713, "Abort If Error"=w712, "Z Correction Active"=w711, "XY Correction Active"=w710, "PID Values"=w700, "Flip XY Axis"=w699, "Invert X Axis"=w698, "Invert Y Axis"=w697, "Invert Z Axis"=w696) -> (w709:T7)
            n105 = control-ref of="This VI"() -> (w707:refnum<vi>)
            n106 = Flatten To JSON(anything=w709) -> (JSON string=w702:string)  [unwired: 2 in, 1 out]
            n107 = property class="VI"(reference=w707) -> ("Path"=w704:path)  [unwired: 1 in, 2 out]
            n108 = Strip Path(path=w704) -> (stripped path=w703:path)  [unwired: 1 out]
            n109 = Build Path(base path=w703, name or relative path="4Pi Objective Lock Default Settings") -> (appended path=w705:path)
            n110 = Build Path(base path=w705, name or relative path="Default Obj Lock Settings.json") -> (appended path=w701:path)
            n111 = Write to Text File(file (use dialog)=w701, text=w702) -> (refnum out=w695:refnum<file>)  [unwired: 2 in, 2 out]
            n112 = Close File(refnum=w695) -> ()  [unwired: 1 in, 2 out]
          }
          event "Start Lock": Value Change {
            n113 = event-data() -> ("NewVal"=w726:bool)  [unwired: 1 in]
            n114 = Select(t=4Pi_Obj_Lock_-_Actions."Start Lock", s=w726, f=4Pi_Obj_Lock_-_Actions."Abort" ("Actions")) -> (s? t:f=w724:T6)
            n115 = Get Notifier Status(notifier=w729) -> (notifier out=w728:refnum<notifier>, current notification=w727:T8)  [unwired: 1 in, 3 out]
            n116 = Bundle By Name(cluster=w727, "Actions"=w724) -> (w723:T8)
            n117 = Send Notification(notification=w723, notifier=w728) -> ()  [unwired: 1 in, 2 out]
          }
          event "Restart Lock": Value Change {
            n118 = event-data() -> ()  [unwired: 1 in, 1 out]
            n119 = Get Notifier Status(notifier=w736) -> (notifier out=w735:refnum<notifier>, current notification=w734:T8)  [unwired: 1 in, 3 out]
            n120 = Bundle By Name(cluster=w734, "Actions"=4Pi_Obj_Lock_-_Actions."Restart Lock" ("t")) -> (w733:T8)
            n121 = local write "Start Lock"(TRUE ("Start Lock")) -> ()
            n122 = Send Notification(notification=w733, notifier=w735) -> ()  [unwired: 1 in, 2 out]
          }
          event "Quit": Value Change {
            # "Turn off the OBJ lock before quiting."
            n123 = event-data() -> ("NewVal"=w747:bool)  [unwired: 1 in]
            n124 = Get Notifier Status(notifier=w742) -> (notifier out=w740:refnum<notifier>, current notification=w738:T8)  [unwired: 1 in, 3 out]
            n125 = Unbundle By Name(w738) -> ("Running?"=w741:bool)
            n126 = case shown="True" w741 {
              tunnel: w740 -> [w748 w752]
              tunnel: [w748 w749] -> w739
              tunnel: w738 -> [_ w754]
              frame False {
              }
              frame True {
                n127 = Bundle By Name(cluster=w754, "Actions"=4Pi_Obj_Lock_-_Actions."Abort") -> (w751:T8)
                n128 = Send Notification(notification=w751, notifier=w752) -> (notifier out=w750:refnum<notifier>)  [unwired: 1 in, 1 out]
                n129 = while {
                  tunnel: w750 -> [w764]
                  tunnel: [w759] -> w749
                  i -> [w758]
                  stop <- w760 stop-if-true
                  n130 = Get Notifier Status(notifier=w764) -> (notifier out=w759:refnum<notifier>, # waiting=w763:i32)  [unwired: 1 in, 3 out]
                  n131 = Greater?(x=w758, y=1500) -> (0:w756:bool)
                  n132 = Less?(x=w763, y=1) -> (x < y?=w761:bool)
                  n133 = Or(x=w761, y=w756) -> (x .or. y?=w760:bool)
                  n134 = Wait (ms)(milliseconds to wait=u32 1) -> ()  [unwired: 1 out]
                }
              }
            }
            n135 = Get Notifier Status(notifier=w739) -> (notifier out=w744:refnum<notifier>, current notification=w746:T8)  [unwired: 1 in, 3 out]
            n136 = Bundle By Name(cluster=w746, "Actions"=4Pi_Obj_Lock_-_Actions."Quit") -> (w743:T8)
            n137 = Send Notification(notification=w743, notifier=w744) -> ()  [unwired: 1 in, 2 out]
          }
        }
      }
      n138 = while {
        tunnel: w150 -> [w176]
        tunnel: w148 -> [w164]
        tunnel: w147 -> [w163]
        tunnel: w149 -> [w175]
        stop <- w171 stop-if-true
        # "Column 1 - Target Lock Values\nColumn 2 - Current Values\nColumn 3 - Differnce Values\nColumn 4 - Initial XYZ Stage Positions"
        n139 = Wait on Notification(notifier=w175, ignore previous (F)=FALSE) -> (notifier out=w170:refnum<notifier>, notification=w173:T8)  [unwired: 2 in, 2 out]
        n140 = Unbundle By Name(w173) -> ("Actions"=w165:T6)
        n141 = Equal?(x=4Pi_Obj_Lock_-_Actions."Quit", y=w165) -> (x = y?=w171:bool)
        n142 = Initialize Array(0.0 ("element"), 3 ("dimension size"), 4 ("dimension size")) -> (w167:dbl[][])
        n143 = while {
          shift-right: [w183] -> _
          shift-left: w165 -> [w191]
          tunnel: w176 -> [w195]
          tunnel: w164 -> [w194]
          tunnel: w163 -> [w193]
          tunnel: w170 -> [w189]
          shift-right: [w177] -> _
          shift-left: w167 -> [w178]
          stop <- w190 stop-if-true
          w185 = 4Pi_Obj_Lock_-_Actions."Abort" ("x")
          n144 = case shown="\"Move XYZ\", \"Move XY\"" w191 {
            selector: w191 -> [_ _ _ _ _ _ w429 _ _ _ _ _ _]
            tunnel: w195 -> [_ w201 w269 w334 w369 _ _ _ _ _ w582 _ _]
            tunnel: w194 -> [_ w210 w244 _ _ _ w433 _ _ _ _ _ _]
            tunnel: w193 -> [_ w209 w243 _ _ _ _ w513 _ _ _ _ _]
            tunnel: FALSE -> [w198 w230 w272 w335 w370 w404 w467 w518 w560 w569 w586 _ _]
            tunnel: [4Pi_Obj_Lock_-_Actions."Exit Loop" ("x") w223 w264 w313 w352 w379 w448 w486 4Pi_Obj_Lock_-_Actions."Delay" ("x") 4Pi_Obj_Lock_-_Actions."Get Current Position" ("x") 4Pi_Obj_Lock_-_Actions."Exit Loop" ("x") 4Pi_Obj_Lock_-_Actions."Exit Loop" ("x") 4Pi_Obj_Lock_-_Actions."Quit" ("x")] -> w184
            tunnel: [w198 w230 w272 w335 w370 w404 w467 w518 w560 w569 w586 TRUE TRUE] -> w190
            tunnel: w189 -> [w197 w229 w271 w333 w368 w403 w466 w516 w558 w567 w590 w596 w600]
            tunnel: [w197 w229 w271 w322 w367 w402 w465 w515 w557 w563 w589 w596 w600] -> w188
            tunnel: w178 -> [w196 w206 w256 w329 w340 w389 w419 w484 w550 w566 w585 w595 w599]
            tunnel: [w196 w205 w255 w328 w339 w386 w419 w484 w550 w566 w585 w595 w599] -> w177
            frame "Idle", Default {
            }
            frame "Start Lock" {
              w200 = FALSE ("Move Limit Error")
              w207 = Stage_Actions."Get Position" ("Actions")
              w222 = T15 [] ("History Data")
              # "Make sure the camera is running, if not abort."
              n145 = control-ref of="This VI"() -> (w220:refnum<vi>)
              n146 = call "Stages Messenger.vi"("Stage Notifier Name"=w210, "Actions"=w207) -> ("Positions"=w211:dbl[])  [unwired: 10 in, 3 out]
              n147 = call "Stages Messenger.vi"("Stage Notifier Name"=w209, "Actions"=w207) -> ("Positions"=w212:dbl[])  [unwired: 10 in, 3 out]
              n148 = property class="VI"(reference=w220) -> ("Path"=w217:path)  [unwired: 1 in, 2 out]
              n149 = Index Array(array=w212, index=0) -> (element=w208:dbl)
              n150 = Strip Path(path=w217) -> (stripped path=w216:path)  [unwired: 1 out]
              n151 = Build Path(base path=w216, name or relative path="4Pi Objective Lock Default Settings") -> (appended path=w218:path)
              n152 = Build Array (concatenate)(w211, w208) -> (w203:dbl[])
              n153 = Build Path(base path=w218, name or relative path="Initial Stage Positions.json") -> (appended path=w214:path)
              n154 = Flatten To JSON(anything=w203) -> (JSON string=w215:string)  [unwired: 2 in, 1 out]
              n155 = Replace Array Subset(array=w206, new element=w203, index (col)=3 ("disabled index (col)")) -> (w205:dbl[][])  [unwired: 1 in]
              n156 = Write to Text File(file (use dialog)=w214, text=w215) -> (refnum out=w202:refnum<file>)  [unwired: 2 in, 2 out]
              n157 = Close File(refnum=w202) -> ()  [unwired: 1 in, 2 out]
              n158 = local write "Move Limit Error"(w200) -> ()
              n159 = local write "Fit Error"(w200) -> ()
              n160 = call "Camera Messenger.vi"("Notifier Name"=w201, "General Camera Actions"=Generic_Camera_Actions."Live Preview") -> ("Notifier Name Dup"=w227:string)  [unwired: 8 in, 5 out]
              n161 = while {
                tunnel: w227 -> [w237]
                tunnel: [w232] -> w226
                i -> [w236]
                stop <- w233 stop-if-true
                n162 = call "Camera Messenger.vi"("Notifier Name"=w237, "General Camera Actions"=Generic_Camera_Actions."Status") -> ("Running?"=w234:bool)  [unwired: 8 in, 5 out]
                n163 = Greater?(x=w236, y=3000) -> (0:w232:bool)
                n164 = Or(x=w234, y=w232) -> (x .or. y?=w233:bool)
                n165 = Wait (ms)(milliseconds to wait=u32 1) -> ()  [unwired: 1 out]
              }
              n166 = property on="X Target and Fit Position (px)" class="WFChart (strict)"("History Data"=w222) -> ()  [unwired: 2 in, 2 out]
              n167 = property on="Y Target and Fit Position (px)" class="WFChart (strict)"("History Data"=w222) -> ()  [unwired: 2 in, 2 out]
              n168 = property on="Z sx/sy Target and Fit Value" class="WFChart (strict)"("History Data"=w222) -> ()  [unwired: 2 in, 2 out]
              n169 = Select(t=4Pi_Obj_Lock_-_Actions."Exit Loop" ("x"), s=w226, f=4Pi_Obj_Lock_-_Actions."Get Initial Position" ("x")) -> (s? t:f=w223:T6)
            }
            frame "Restart Lock" {
              w239 = FALSE ("Move Limit Error")
              w263 = T15 [] ("History Data")
              # "Make sure the camera is running, if not abort."
              n170 = control-ref of="This VI"() -> (w261:refnum<vi>)
              n171 = call "Camera Messenger.vi"("Notifier Name"=w269, "General Camera Actions"=Generic_Camera_Actions."Live Preview") -> ("Notifier Name Dup"=w268:string)  [unwired: 8 in, 5 out]
              n172 = property class="VI"(reference=w261) -> (error out=w247:errorcluster, "Path"=w258:path)  [unwired: 1 in, 1 out]
              n173 = while {
                tunnel: w268 -> [w298]
                tunnel: [w293] -> w267
                i -> [w297]
                stop <- w294 stop-if-true
                n174 = call "Camera Messenger.vi"("Notifier Name"=w298, "General Camera Actions"=Generic_Camera_Actions."Status") -> ("Running?"=w295:bool)  [unwired: 8 in, 5 out]
                n175 = Greater?(x=w297, y=3000) -> (0:w293:bool)
                n176 = Or(x=w295, y=w293) -> (x .or. y?=w294:bool)
                n177 = Wait (ms)(milliseconds to wait=u32 1) -> ()  [unwired: 1 out]
              }
              n178 = Strip Path(path=w258) -> (stripped path=w257:path)  [unwired: 1 out]
              n179 = Build Path(base path=w257, name or relative path="4Pi Objective Lock Default Settings") -> (appended path=w259:path)
              n180 = Build Path(base path=w259, name or relative path="Initial Stage Positions.json") -> (appended path=w253:path)
              n181 = Read from Text File(file (use dialog)=w253, error in=w247) -> (refnum out=w252:refnum<file>, text=w251:string, error out=w250:errorcluster)  [unwired: 2 in, 1 out]
              n182 = Close File(refnum=w252, error in=w250) -> (error out=w249:errorcluster)  [unwired: 1 out]
              n183 = local write "Move Limit Error"(w239) -> ()
              n184 = local write "Fit Error"(w239) -> ()
              n185 = Unflatten From JSON(JSON string=w251, type and defaults=dbl[] [], error in (no error)=w249) -> (value=w245:dbl[], error out=w246:errorcluster)  [unwired: 4 in]
              n186 = case shown="Error" w246 {
                tunnel: w245 -> [w274 _]
                tunnel: w244 -> [w281 w286]
                tunnel: w243 -> [w280 w285]
                tunnel: [w274 w284] -> w242
                tunnel: u32 150 ("milliseconds to wait") -> [w273 w283]
                tunnel: [w273 w283] -> w240
                frame No Error {
                  w282 = Stage_Actions."MOVE" ("Actions")
                  n187 = Split 1D Array(array=w274, index=2) -> (first subarray=w278:dbl[], second subarray=w277:dbl[])
                  n188 = call "Stages Messenger.vi"("Stage Notifier Name"=w281, "Actions"=w282, "Setpoint"=w278, "Axis"=bool[] [TRUE, TRUE]) -> ()  [unwired: 8 in, 4 out]
                  n189 = call "Stages Messenger.vi"("Stage Notifier Name"=w280, "Actions"=w282, "Setpoint"=w277, "Axis"=bool[] [TRUE]) -> ()  [unwired: 8 in, 4 out]
                }
                frame Error {
                  w287 = Stage_Actions."Get Position" ("Actions")
                  n190 = call "Stages Messenger.vi"("Stage Notifier Name"=w286, "Actions"=w287) -> ("Positions"=w289:dbl[])  [unwired: 10 in, 3 out]
                  n191 = call "Stages Messenger.vi"("Stage Notifier Name"=w285, "Actions"=w287) -> ("Positions"=w290:dbl[])  [unwired: 10 in, 3 out]
                  n192 = Index Array(array=w290, index=0) -> (element=w288:dbl)
                  n193 = Build Array (concatenate)(w289, w288) -> (w284:dbl[])
                }
              }
              n194 = Wait (ms)(milliseconds to wait=w240) -> ()  [unwired: 1 out]
              n195 = property on="X Target and Fit Position (px)" class="WFChart (strict)"("History Data"=w263) -> ()  [unwired: 2 in, 2 out]
              n196 = property on="Y Target and Fit Position (px)" class="WFChart (strict)"("History Data"=w263) -> ()  [unwired: 2 in, 2 out]
              n197 = property on="Z sx/sy Target and Fit Value" class="WFChart (strict)"("History Data"=w263) -> ()  [unwired: 2 in, 2 out]
              n198 = Replace Array Subset(array=w256, new element=w242, index (col)=3 ("disabled index (col)")) -> (w255:dbl[][])  [unwired: 1 in]
              n199 = Select(t=4Pi_Obj_Lock_-_Actions."Exit Loop" ("x"), s=w267, f=4Pi_Obj_Lock_-_Actions."Get Initial Position" ("x")) -> (s? t:f=w264:T6)
            }
            frame "Get Initial Position" {
              w306 = 0 ("index")
              # "Set target values"
              n200 = Get Notifier Status(notifier=w333) -> (notifier out=w323:refnum<notifier>, current notification=w321:T8)  [unwired: 1 in, 3 out]
              n201 = Unbundle By Name(w321) -> ("Frame Accumulations"=w332:u16)
              n202 = Bundle By Name(cluster=w321, "Running?"=TRUE) -> (w319:T8)
              n203 = Send Notification(notification=w319, notifier=w323) -> (notifier out=w322:refnum<notifier>)  [unwired: 1 in, 1 out]
              n204 = call "Generic Camera Get New Camera Image.vi"("Camera Notifier Name"=w334, "Frames"=w332) -> ("Image - U16"=w331:u16[][], "Error"=w330:errorcluster)  [unwired: 11 in, 1 out]
              n205 = call "2D Gaussian - Fit Image U16.vi"("Image In (U16)"=w331, "Error In"=w330) -> ("Best Fit Params"=w327:T16, "Error Out"=w312:errorcluster)  [unwired: 12 in]
              n206 = Unbundle By Name(w312) -> ("status"=w311:bool)
              n207 = Cluster To Array(cluster=w327) -> (array=w326:dbl[])
              n208 = local write "Fit Error"(w311) -> ()
              n209 = Array Subset(array=w326, index=1, length=4) -> (w318:dbl[])
              n210 = Index Array(array=w318, index #1=0 ("index"), index #2=1 ("index"), index #3=2 ("index"), index #4=3 ("index")) -> (element #1=w300:dbl, element #2=w301:dbl, element #3=w308:dbl, element #4=w307:dbl)
              "Target X Position (px)" <- w300
              "Target Y Position (px)" <- w301
              n211 = Divide(x=w308, y=w307) -> (x/y=w302:dbl)
              "Target sx/sy" <- w302
              n212 = Replace Array Subset(array=w329, new element #1=w300, index (row) #1=0 ("disabled index (row)"), index (col) #1=w306, new element #2=w301, index (row) #2=1 ("disabled index (row)"), index (col) #2=w306, new element #3=w302, index (row) #3=2 ("disabled index (row)"), index (col) #3=w306) -> (w328:dbl[][])
              n213 = Select(t=4Pi_Obj_Lock_-_Actions."Abort" ("x"), s=w311, f=4Pi_Obj_Lock_-_Actions."Get Current Position" ("x")) -> (s? t:f=w313:T6)
            }
            frame "Get Current Position" {
              w344 = 1 ("index")
              # "Update current values"
              n214 = Get Notifier Status(notifier=w368) -> (notifier out=w367:refnum<notifier>, current notification=w366:T8)  [unwired: 1 in, 3 out]
              n215 = Unbundle By Name(w366) -> ("Abort If Error"=w357:bool, "Frame Accumulations"=w365:u16)
              n216 = call "Generic Camera Get New Camera Image.vi"("Camera Notifier Name"=w369, "Frames"=w365) -> ("Image - U16"=w364:u16[][], "Error"=w363:errorcluster)  [unwired: 11 in, 1 out]
              n217 = call "2D Gaussian - Fit Image U16.vi"("Image In (U16)"=w364, "Error In"=w363) -> ("Best Fit Params"=w362:T16, "Error Out"=w358:errorcluster)  [unwired: 12 in]
              n218 = Unbundle By Name(w358) -> ("status"=w356:bool)
              "Fit Error" <- w356
              n219 = And(x=w357, y=w356) -> (x .and. y?=w355:bool)
              n220 = Cluster To Array(cluster=w362) -> (array=w361:dbl[])
              n221 = Array Subset(array=w361, index=1, length=4) -> (w345:dbl[])
              n222 = Index Array(array=w345, index #1=0 ("index"), index #2=1 ("index"), index #3=2 ("index"), index #4=3 ("index")) -> (element #1=w336:dbl, element #2=w337:dbl, element #3=w347:dbl, element #4=w346:dbl)
              "Measured X Position (px)" <- w336
              "Measured Y Position (px)" <- w337
              n223 = Divide(x=w347, y=w346) -> (x/y=w338:dbl)
              "Measured sx/sy" <- w338
              n224 = Select(t=4Pi_Obj_Lock_-_Actions."Abort" ("x"), s=w355, f=4Pi_Obj_Lock_-_Actions."Check Drift" ("x")) -> (s? t:f=w352:T6)
              n225 = Replace Array Subset(array=w340, new element #1=w336, index (row) #1=0 ("disabled index (row)"), index (col) #1=w344, new element #2=w337, index (row) #2=1 ("disabled index (row)"), index (col) #2=w344, new element #3=w338, index (row) #3=2 ("disabled index (row)"), index (col) #3=w344) -> (w339:dbl[][])
            }
            frame "Check Drift" {
              # "Update the PID difference between target values and current values"
              # "Check if Sigma X / Sigma Y is over the limit"
              # "Check if XY values are over the limit"
              n226 = Get Notifier Status(notifier=w403) -> (notifier out=w402:refnum<notifier>, current notification=w401:T8)  [unwired: 1 in, 3 out]
              n227 = Unbundle By Name(w401) -> ("Z Correction Active"=w375:bool, "XY Correction Active"=w377:bool, "XY Drift Threshold"=w397:dbl, "Z Drift Threshold"=w396:dbl, "PID Values"=w400:dbl[])
              n228 = Index Array(array=w389, index (col) #1=0 ("disabled index (col)"), index (col) #2=1 ("index (col)")) -> (element #1=w391:dbl[], element #2=w390:dbl[])  [unwired: 2 in]
              n229 = Array To Cluster(array=w400) -> (cluster=w399:T17)
              n230 = Build Array(w399) -> (w398:T18)
              n231 = call-poly <vilib>:"PID.vi"("PID gains"=w398, "process variable"=w390, "setpoint"=w391) -> ("output"=w387:dbl[])  [unwired: 7 in, 1 out]
              n232 = Build Array(w397, w397, w396) -> (w394:dbl[])
              n233 = Absolute Value(x=w387) -> (abs(x)=w395:dbl[])
              n234 = Replace Array Subset(array=w389, new element=w387, index (col)=2 ("disabled index (col)")) -> (w386:dbl[][])  [unwired: 1 in]
              n235 = Greater?(x=w395, y=w394) -> (0:w385:bool[])
              n236 = Split 1D Array(array=w385, index=2) -> (first subarray=w383:bool[], second subarray=w382:bool[])
              n237 = Or Array Elements(Boolean array=w383) -> (logical OR=w378:bool)
              n238 = Or Array Elements(Boolean array=w382) -> (logical OR=w374:bool)
              n239 = And(x=w377, y=w378) -> (x .and. y?=w376:bool)
              n240 = And(x=w375, y=w374) -> (x .and. y?=w373:bool)
              n241 = Build Array(w376, w373) -> (w381:bool[])
              n242 = Boolean Array To Number(Boolean array=w381) -> (number=w380:u32)
              n243 = case shown="2" w380 {
                tunnel: [4Pi_Obj_Lock_-_Actions."Update Plots" ("x") 4Pi_Obj_Lock_-_Actions."Move XY" ("x") 4Pi_Obj_Lock_-_Actions."Move Z" ("x") 4Pi_Obj_Lock_-_Actions."Move XYZ" ("x")] -> w379
                tunnel: [w405 TRUE FALSE w413] -> w372
                tunnel: [w405 FALSE TRUE w413] -> w371
                frame 0, Default {
                  w405 = FALSE
                  # "XYZ within limits, no move"
                }
                frame 1 {
                  # "X or Y outside limit, move XY"
                }
                frame 2 {
                  # "Sigma X / Y outside limit, move Z"
                }
                frame 3 {
                  w413 = FALSE
                  # "XYZ outside limit, move all"
                }
              }
              "XY Move" <- w372
              "Z Move" <- w371
            }
            frame "Move XYZ", "Move XY" {
              w441 = 2.0
              # "Initial XY stage positions"
              # "Column 3"
              # "Row 1"
              # "Check if move will go beyond ±2 µm of the original positions"
              # "Get XY Diff Values"
              n244 = Get Notifier Status(notifier=w466) -> (notifier out=w465:refnum<notifier>, current notification=w464:T8)  [unwired: 1 in, 3 out]
              n245 = Unbundle By Name(w464) -> ("Abort If Error"=w449:bool, "XY Stage Move Limit (µm)"=w452:dbl)
              n246 = Array Subset(array=w419, index (row)=0 ("index"), length (row)=2 ("length"), index (col)=2 ("index")) -> (w459:dbl[][])  [unwired: 1 in]
              n247 = Array Subset(array=w419, index (row)=0 ("index"), length (row)=2 ("length"), index (col)=3 ("index"), length (col)=1 ("length")) -> (w418:dbl[][])
              n248 = Index Array(array=w459, index (col)=0 ("disabled index (col)")) -> (element=w458:dbl[])  [unwired: 1 in]
              n249 = Index Array(array=w418, index (col)=0 ("disabled index (col)")) -> (element=w416:dbl[])  [unwired: 1 in]
              n250 = Equal?(x=4Pi_Obj_Lock_-_Actions."Move XYZ", y=w429) -> (x = y?=w427:bool)
              n251 = call "4Pi Obj Lock - Rotate Flip XY.vi"("XY Amounts"=w458, "Flip XY"="Flip XY Axis", "Invert X"="Invert X Axis", "Invert Y"="Invert Y Axis") -> ("45° Rotated XY"=w454:dbl[])  [unwired: 11 in]
              n252 = call "Stages Messenger.vi"("Stage Notifier Name"=w433, "Actions"=Stage_Actions."Get Position") -> ("Stage Notifier Name (Dup)"=w432:string, "Positions"=w431:dbl[])  [unwired: 10 in, 2 out]
              n253 = Multiply(x=w454, y=0.005) -> (x*y=w415:dbl[])
              n254 = Add(x=w431, y=w415) -> (x+y=w430:dbl[])
              n255 = Select(t=4Pi_Obj_Lock_-_Actions."Move Z" ("x"), s=w427, f=4Pi_Obj_Lock_-_Actions."Update Plots") -> (s? t:f=w424:T6)
              n256 = Add(x=w416, y=w441) -> (x+y=w439:dbl[])
              n257 = Subtract(x=w416, y=w441) -> (x-y=w440:dbl[])
              n258 = Absolute Value(x=w415) -> (abs(x)=w451:dbl[])
              n259 = Greater?(x=w452, y=w451) -> (0:w450:bool[])
              n260 = In Range and Coerce(upper limit=w439, x=w430, lower limit=w440) -> (In Range?=w438:bool[])  [unwired: 1 out]
              n261 = And Array Elements(Boolean array=w450) -> (logical AND=w437:bool)
              n262 = And Array Elements(Boolean array=w438) -> (logical AND=w435:bool)
              n263 = And(x=w437, y=w435) -> (x .and. y?=w436:bool)
              n264 = Not(x=w436) -> (.not. x?=→"Move Limit Error":bool)
              n265 = case shown="True" w436 {
                tunnel: w415 -> [_ w476]
                tunnel: w449 -> [w472 _]
                tunnel: [w470 w473] -> w448
                tunnel: w432 -> [_ w475]
                tunnel: [dbl[] [-1.0, -1.0] ("Positions") w474] -> w446
                tunnel: w424 -> [w468 w473]
                frame False {
                  n266 = Select(t=4Pi_Obj_Lock_-_Actions."Abort" ("x"), s=w472, f=w468) -> (s? t:f=w470:T6)
                }
                frame True {
                  n267 = call "Stages Messenger.vi"("Stage Notifier Name"=w475, "Actions"=Stage_Actions."MVR", "Setpoint"=w476, "Axis"=bool[] [TRUE, TRUE]) -> ("Positions"=w474:dbl[])  [unwired: 8 in, 3 out]
                }
              }
              n268 = Index Array(array=w446, index #1=0 ("index"), index #2=1 ("index")) -> (element #1=→"X Axis Position (µm)":dbl, element #2=→"Y Axis Position (µm)":dbl)
            }
            frame "Move Z" {
              w491 = 2.0 ("y")
              w503 = 0 ("disabled index (col)")
              # "Initial Z stage position"
              # "Get sx/sy Diff Value"
              n269 = Get Notifier Status(notifier=w516) -> (notifier out=w515:refnum<notifier>, current notification=w517:T8)  [unwired: 1 in, 3 out]
              n270 = Index Array(array=w484, index (row)=2, index (col)=3 ("disabled index (col)")) -> (element=w481:dbl)
              n271 = Unbundle By Name(w517) -> ("Abort If Error"=w490:bool, "Z Stage Move Limit (µm)"=w495:dbl)
              n272 = Array Subset(array=w484, index (row)=2 ("index"), length (row)=1 ("length"), index (col)=2 ("index"), length (col)=1 ("length")) -> (w507:dbl[][])
              n273 = Index Array(array=w507, index (row)=w503, index (col)=w503) -> (element=w504:dbl)
              n274 = Multiply(x=w504, y=-1.0) -> (x*y=w500:dbl)
              n275 = Add(x=w481, y=w491) -> (x+y=w497:dbl)
              n276 = Subtract(x=w481, y=w491) -> (x-y=w496:dbl)
              n277 = call "Stages Messenger.vi"("Stage Notifier Name"=w513, "Actions"=Stage_Actions."Get Position") -> ("Stage Notifier Name (Dup)"=w492:string, "Positions"=w511:dbl[])  [unwired: 10 in, 2 out]
              n278 = Negate(x=w500) -> (-x=w501:dbl)
              n279 = Select(t=w501, s="Invert Z Axis", f=w500) -> (s? t:f=w487:dbl)
              n280 = Index Array(array=w511, index=0) -> (element=w502:dbl)
              n281 = Greater?(x=w495, y=w487) -> (0:w494:bool)
              n282 = Add(x=w487, y=w502) -> (x+y=w498:dbl)
              n283 = In Range and Coerce(upper limit=w497, x=w498, lower limit=w496) -> (In Range?=w493:bool)  [unwired: 1 out]
              n284 = Multiply(x=0.3, y=w487) -> (x*y=w480:dbl)
              n285 = And(x=w494, y=w493) -> (x .and. y?=w489:bool)
              n286 = Not(x=w489) -> (.not. x?=w488:bool)
              n287 = case shown="True" w489 {
                tunnel: w492 -> [_ w531]
                tunnel: w490 -> [w522 _]
                tunnel: w480 -> [_ w530]
                tunnel: [w521 4Pi_Obj_Lock_-_Actions."Update Plots" ("x")] -> w486
                tunnel: [-1.0 ("Position") w525] -> w485
                frame False {
                  n288 = Select(t=4Pi_Obj_Lock_-_Actions."Abort" ("x"), s=w522, f=4Pi_Obj_Lock_-_Actions."Update Plots") -> (s? t:f=w521:T6)
                }
                frame True {
                  n289 = Build Array(w530) -> (w529:dbl[])
                  n290 = call "Stages Messenger.vi"("Stage Notifier Name"=w531, "Actions"=Stage_Actions."MVR", "Setpoint"=w529, "Axis"=bool[] [TRUE]) -> ("Positions"=w527:dbl[])  [unwired: 8 in, 3 out]
                  n291 = Index Array(array=w527, index=0) -> (element=w525:dbl)
                }
              }
              "Z Axis Position (µm)" <- w485
              n292 = local write "Move Limit Error"(w488) -> ()
            }
            frame "Update Plots" {
              w549 = 1 ("index (row)")
              w555 = 0 ("index (row)")
              # "This is all a bit messy..."
              # "Current Values"
              # "Target Values"
              n293 = Get Notifier Status(notifier=w558) -> (notifier out=w557:refnum<notifier>, current notification=w559:T8)  [unwired: 1 in, 3 out]
              n294 = Unbundle By Name(w559) -> ("Z Drift Threshold"=w544:dbl, "XY Drift Threshold"=w542:dbl, "PID Values"=w546:dbl[])
              n295 = Index Array(array=w550, index (row) #1=0 ("index (row)"), index (col) #1=w549, index (row) #2=1 ("index (row)"), index (col) #2=w549, index (row) #3=2 ("disabled index (row)"), index (col) #3=w549) -> (element #1=w539:dbl, element #2=w534:dbl, element #3=w548:dbl)
              n296 = Index Array(array=w550, index (row) #1=w555, index (col) #1=w555, index (row) #2=1 ("index (row)"), index (col) #2=w555, index (row) #3=2 ("disabled index (row)"), index (col) #3=w555) -> (element #1=w540:dbl, element #2=w536:dbl, element #3=w533:dbl)
              n297 = Index Array(array=w546, index=0) -> (element=w541:dbl)
              n298 = Divide(x=w542, y=w541) -> (x/y=w537:dbl)
              n299 = call "4Pi Obj Lock - 1 Values Organize Plot Data.vi"("Target 01"=w536, "Value Limit"=w537, "Current 01"=w534) -> ("Plot Data"=→"Y Target and Fit Position (px)":T2)  [unwired: 12 in]
              n300 = Divide(x=w544, y=w541) -> (x/y=w543:dbl)
              n301 = call "4Pi Obj Lock - 1 Values Organize Plot Data.vi"("Target 01"=w540, "Value Limit"=w537, "Current 01"=w539) -> ("Plot Data"=→"X Target and Fit Position (px)":T2)  [unwired: 12 in]
              n302 = call "4Pi Obj Lock - 1 Values Organize Plot Data.vi"("Target 01"=w533, "Value Limit"=w543, "Current 01"=w548) -> ("Plot Data"=→"Z sx/sy Target and Fit Value":T2)  [unwired: 12 in]
            }
            frame "Delay" {
              n303 = Get Notifier Status(notifier=w567) -> (notifier out=w565:refnum<notifier>, current notification=w568:T8)  [unwired: 1 in, 3 out]
              n304 = Unbundle By Name(w568) -> ("Update Delay (ms)"=w564:i32)
              n305 = while {
                tunnel: w565 -> [w580]
                tunnel: w564 -> [w577]
                tunnel: [w573] -> w563
                i -> [w578]
                stop <- w571 stop-if-true
                n306 = Get Notifier Status(notifier=w580) -> (notifier out=w573:refnum<notifier>, current notification=w576:T8)  [unwired: 1 in, 3 out]
                n307 = Greater Or Equal?(x=w578, y=w577) -> (x >= y?=w572:bool)
                n308 = Wait (ms)(milliseconds to wait=u32 1) -> ()  [unwired: 1 out]
                n309 = Unbundle By Name(w576) -> ("Actions"=w575:T6)
                n310 = Equal?(x=w575, y=4Pi_Obj_Lock_-_Actions."Abort") -> (x = y?=w570:bool)
                n311 = Or(x=w570, y=w572) -> (x .or. y?=w571:bool)
              }
            }
            frame "Abort" {
              w584 = 0.0 ("Target X Position (px)")
              n312 = Get Notifier Status(notifier=w590) -> (notifier out=w594:refnum<notifier>, current notification=w593:T8)  [unwired: 1 in, 3 out]
              n313 = call "Camera Messenger.vi"("Notifier Name"=w582, "General Camera Actions"=Generic_Camera_Actions."Abort") -> ()  [unwired: 8 in, 6 out]
              n314 = Bundle By Name(cluster=w593, "Running?"=FALSE, "Actions"=4Pi_Obj_Lock_-_Actions."Exit Loop") -> (w591:T8)
              n315 = Send Notification(notification=w591, notifier=w594) -> (notifier out=w589:refnum<notifier>)  [unwired: 1 in, 1 out]
              n316 = local write "Start Lock"(FALSE ("Start Lock")) -> ()
              n317 = local write "Target X Position (px)"(w584) -> ()
              n318 = local write "Target Y Position (px)"(w584) -> ()
              n319 = local write "Measured X Position (px)"(w584) -> ()
              n320 = local write "Measured Y Position (px)"(w584) -> ()
              n321 = local write "Target sx/sy"(w584) -> ()
              n322 = local write "Measured sx/sy"(w584) -> ()
            }
            frame "Exit Loop" {
            }
            frame "Quit" {
              n323 = Release Notifier(notifier=w600, force destroy? (F)=TRUE) -> ()  [unwired: 1 in, 3 out]
            }
          }
          n324 = Get Notifier Status(notifier=w188) -> (current notification=w187:T8, error out=w182:errorcluster)  [unwired: 1 in, 3 out]
          n325 = Unbundle By Name(w187) -> ("Actions"=w186:T6)
          n326 = Unbundle By Name(w182) -> ("status"=w180:bool)
          n327 = Equal?(x=w185, y=w186) -> (x = y?=w181:bool)
          n328 = Or(x=w181, y=w180) -> (x .or. y?=w179:bool)
          n329 = Select(t=w185, s=w179, f=w184) -> (s? t:f=w183:T6)
        }
      }
      n330 = local write "Quit"(w162) -> ()
    }
    frame Error {
    }
  }
  n331 = control-ref of="This VI"() -> (w69:refnum<vi>)
  n332 = property class="VI"(reference=w69) -> (reference out=w78:refnum<vi>, "Panel"=w70:refnum<vi>)  [unwired: 1 in, 1 out]
  n333 = property class="Pnl"(reference=w70) -> ("Decos[]"=w68:refnum<vi>[], "Panes[]"=w74:refnum<vi>[])  [unwired: 1 in, 2 out]
  n334 = Array Size(array=w68) -> (size(s)=w66:i32)
  n335 = Decrement(x=w66) -> (x-1=w67:i32)
  n336 = Index Array(array=w74, index=0) -> (element=w73:refnum<vi>)
  n337 = Index Array(array=w68, index=w67) -> (element=w76:refnum<vi>)
  n338 = property class="VI"(reference=w78) -> (reference out=w80:refnum<vi>, "Front Panel.PanelBounds"=w81:T19)  [unwired: 1 in, 1 out]
  n339 = property class="Decor"(reference=w76) -> ("Bounds"=w79:T20)  [unwired: 1 in, 2 out]
  n340 = property class="Pane"(reference=w73, "Origin"=T10 {"Horizontal"=0, "Vertical"=0}, "HorizScrollbarVisibility"=w77, "VertScrollbarVisibility"=w77) -> ()  [unwired: 1 in, 2 out]
  n341 = Unbundle By Name(w79) -> ("Width"=w84:u32, "Height"=w87:u32)
  n342 = control-ref of="Quit"() -> (w71:refnum<vi>)
  n343 = To Word Integer(number=w84) -> (16bit integer=w86:i16)
  n344 = To Word Integer(number=w87) -> ()  [unwired: 1 out]
  n345 = property class="Bool (strict)"(reference=w71) -> ("Height"=w89:u32, "Top"=w90:i32)  [unwired: 1 in, 2 out]
  n346 = Unbundle By Name(w81) -> ("Left"=w83:i16, "Top"=w94:i16)
  n347 = To Word Integer(number=w89) -> (16bit integer=w92:i16)
  n348 = To Word Integer(number=w90) -> (16bit integer=w93:i16)
  n349 = Add(x=w83, y=w86) -> (x+y=w85:i16)
  n350 = Compound Arithmetic op=ADD(w94, w92, w93, i16 12 ("y")) -> (w88:i16)
  n351 = Bundle By Name(cluster=w81, "Right"=w85, "Bottom"=w88) -> (w82:T19)
  n352 = property class="VI"(reference=w80, "Front Panel.PanelBounds"=w82) -> ()  [unwired: 1 in, 2 out]
